vi "CRYGraph Wave Window.vi"() -> ()   [LabVIEW 2013]
uses:
  <vilib>/Utility/miscctls.llb/LVPoint32TypeDef.ctl
  Control/CRYFlag Cluster.ctl
  <vilib>/Utility/miscctls.llb/LVRowAndColumnTypeDef.ctl
  <vilib>/Utility/miscctls.llb/LVRectTypeDef.ctl
  CRYCurveLibrary/Global/CRYCurve Library Global.vi
  SubVI/CRYData View Global.vi
  SubVI/CRYMain Sub Window Global.vi
panel:
  out "LegendVScrollShow":bool=TRUE
  out "Legend Ref":refnum<vi>
  out "SelectedRow":i32[](array[numeric])
  in  "LoadFinish":bool
  in  "WhichKey":string
  out "KeyRepeatCount":i32
  in  "CursorMoveFinish":bool
  in  "ScaleFitY 2":bool
  in  "ScaleFitY":bool
  in  "ScaleFitX":bool
  in  "ToolbarUpdate":bool
  out "PropertyTab":string
  in  "OpenProperty":bool
  in  "PaletteShow":bool
  in  "FitPanes":bool
  out "PreviewScaleMax":dbl
  out "PreviewScaleMin":dbl
  out "PreviewCoords":T1
  in  "ScaleRange":bool
  out "Repaint Watermark":i32
  out "Event Name":string
  out "ReportDrop":bool
  out "DirectionKey":bool
  out "PreviewGraph Ref":refnum<vi>
  out "Graph Ref":refnum<vi>
  in  "AxisChange":bool
  in  "RemoveSome":bool
  out "ChildIntensityVI Ref":refnum<vi>
  in  "IntensityShow":bool
  out "ScaleMin":dbl
  out "ScaleMax":dbl
  out "ScrollTick Ref":refnum<vi>
  out "Scrollbar Ref":refnum<vi>
  in  "PreviewShow":bool
  in  "RemoveAll":bool
  in  "CursorColor":bool
  out "NewCursIdx":u32
  out "Test":string
  in  "OldCursIdx":u32
  out "Queue Name":string
  in  "StateOut":bool
  in  "Cursor Waves":string[](array[string])
  out "Cursor Coords":T1
  in  "CursorPlot":bool
  out "Cursor Ref":refnum<vi>
  in  "CursorShow":bool
  out "WaveGraph":cluster{"xo":dbl, "dx":dbl, dbl[]}[](graph)
  out "Title Name":string
  out "OldRow":i32
  out "TotalPlot":u32
  out "Graph Number":i32
  in  "stop":bool
  out "PreviewGraph":cluster{"xo":dbl, "dx":dbl, dbl[]}[](graph)
  in  "CursorEnabled":bool
  in  "Scrollbar":dbl(c297)
  in  "ScrollTick":dbl(slide) scale=0.0..1.0 scale format="%-#3.2p"
  in  "Cursor":string[][](table)
  in  "LegendShow":bool
  in  "ColorBox":u32(colorbox)
  in  "Legend":i32[](listbox)
  in  "GraphType":string
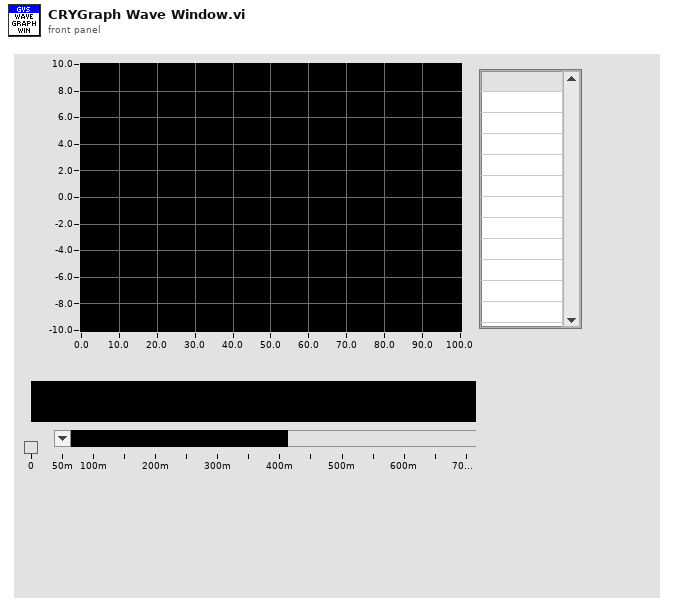
[diagram p1: front panel]
types:
  T1 = typedef "LVPoint32TypeDef.ctl" = cluster{"Horizontal":i32, "Vertical":i32}
  T2 = typedef "CRYFlag Cluster.ctl" = cluster{"LegendShow":bool, "CellClick":bool, "Total Number":bool, "ScaleFitX":bool, "ScaleFitY":bool, "MapModeX":u8, "MapModeY":u8, "CursorShow":bool, "MagnitudeShow":bool, "PreviewShow":bool, "CursorEnabled":bool, "IntensityShow":bool, "PaletteShow":bool, "PhaseShow":bool, "XYShow":bool, "FrequencyShow":bool, "LegendVScrollShow":bool, "FrequencyVScrollShow":bool}
  T3 = typedef "CRYGraph Event.ctl" = cluster{"EvenName":string, "TitleName":string, "GraphName":string, "GraphType":string, "Data":variant, "Queue Name":string, "DataView Number":i32}
  T4 = enum16{"No Scaling", "Scale All Objects", "Scale Single Object"}
  T5 = typedef "LVRowAndColumnTypeDef.ctl" = cluster{"Row":i32, "Column":i32}
  T6 = typedef "LVRectTypeDef.ctl" = cluster{"Left":i16, "Top":i16, "Right":i16, "Bottom":i16}
  T7 = typedef "LVBoundsTypeDef.ctl" = cluster{"Width":u32, "Height":u32}
  T8 = typedef "LVPositionTypeDef.ctl" = cluster{"Left":i32, "Top":i32}
  T9 = typedef "CRYWaveform Cluster.ctl" = cluster{"Waveform":cluster{"X0":dbl, "dX":dbl, "Y":sgl[]}, "X data":u16, "Y data":u16, "Y axis":u16, "X unit":string, "Y unit":string, "Y dB ref":dbl, "display Y":bool, "display X":bool, "Overload?":bool, "Test Info":string, "Step No.":i32, "Name":string, "protected":bool, "Sqc history":string[], "Signal Channel ID":i32, "Plot Settings":cluster{"Color":u32, "Interpolation":u8, "Point Style":u8, "Line Style":u8, "Point Color":u32, "Line Width":u8, "Bar Plot Style":u8, "Fill To":i16}, "AutoProtect":bool}
  T10 = typedef "LVRangeTypeDef.ctl" = cluster{"Minimum":dbl, "Maximum":dbl, "Increment":dbl, "Minor Increment":dbl, "Start":dbl}
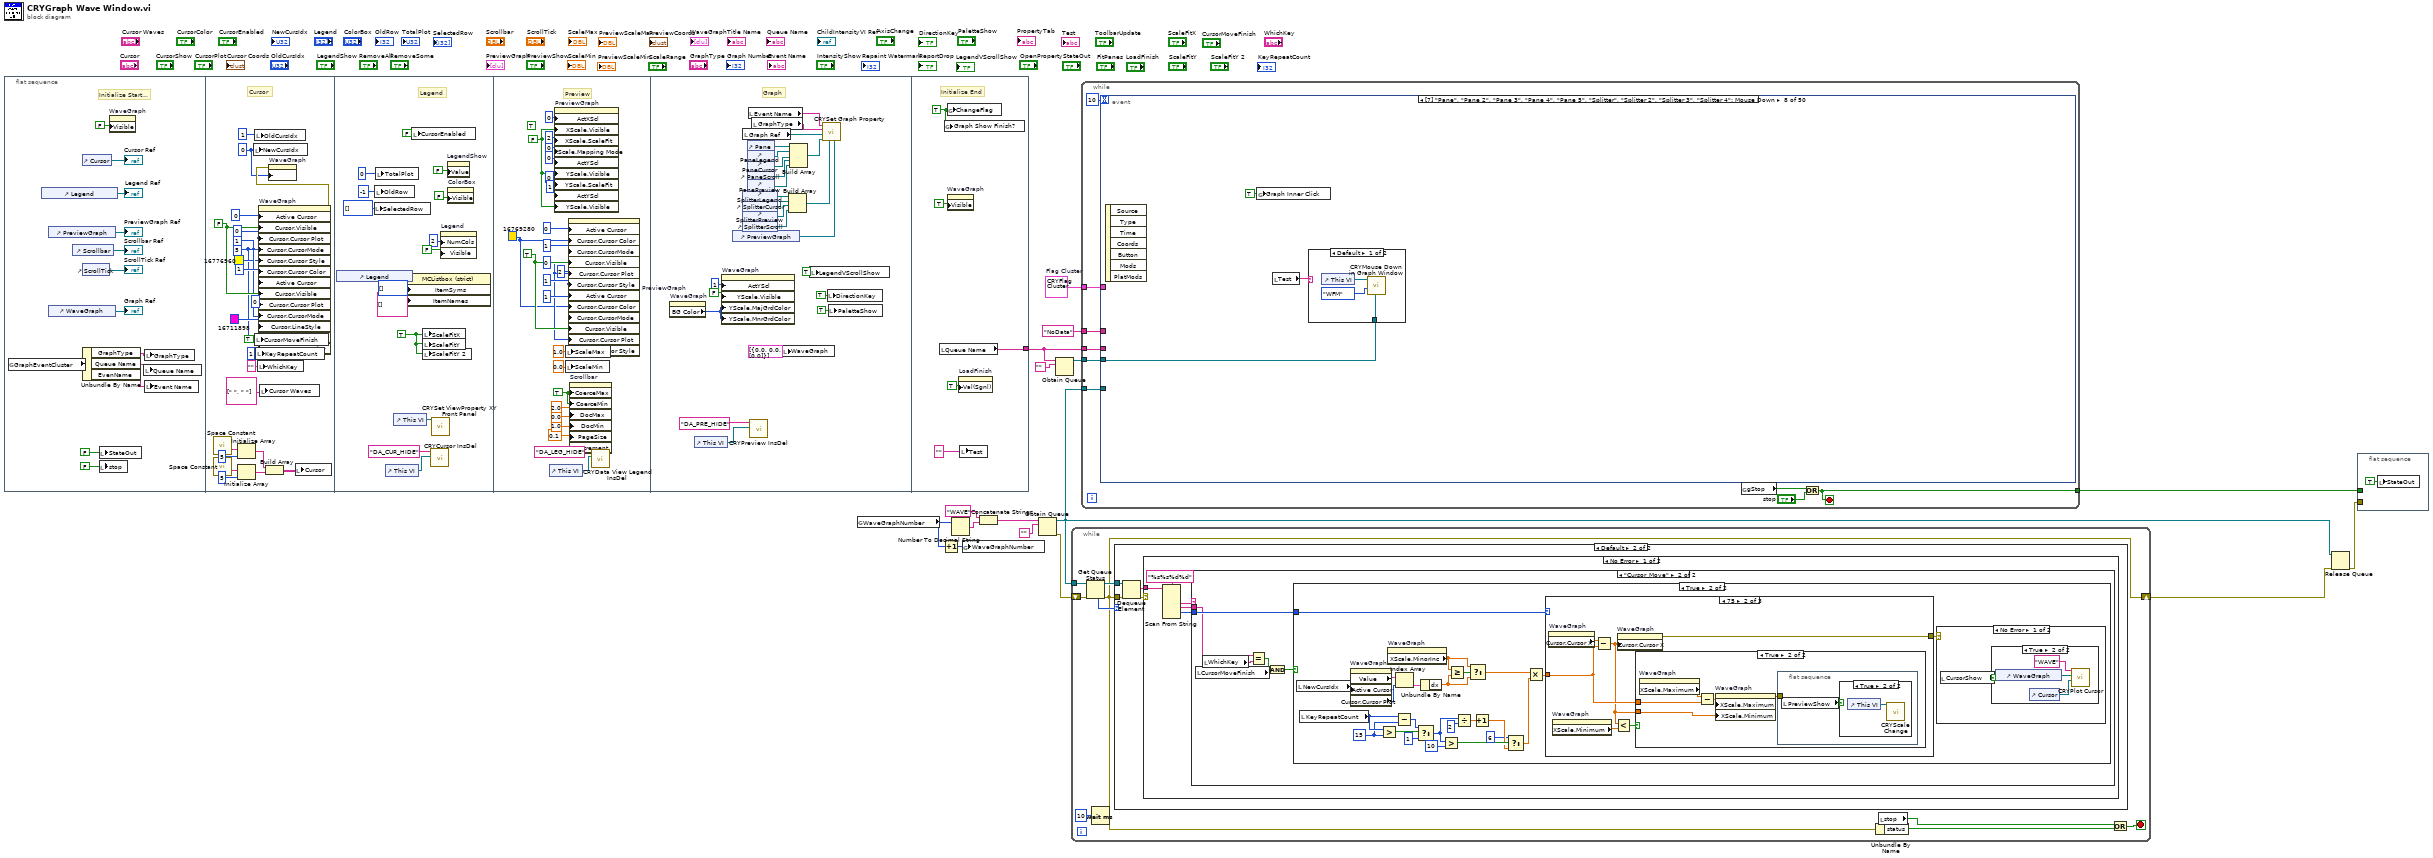
[diagram p0: block diagram]
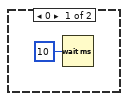
[diagram p2: hidden frame]
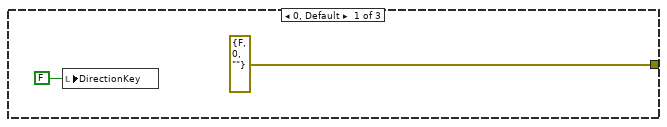
[diagram p7: hidden frame]
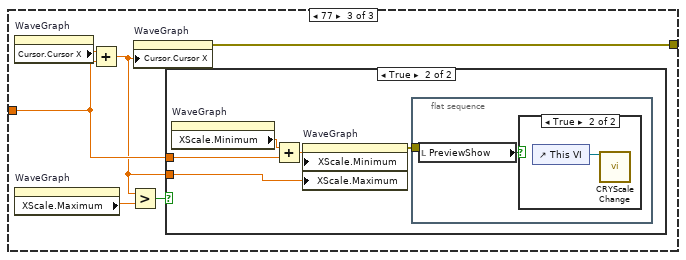
[diagram p10: hidden frame]
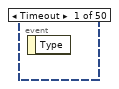
[diagram p14: hidden frame]
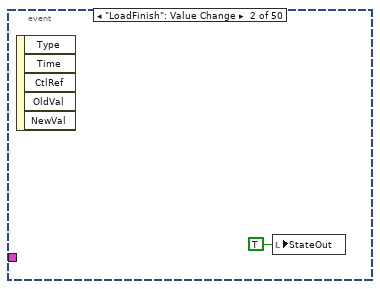
[diagram p15: hidden frame]
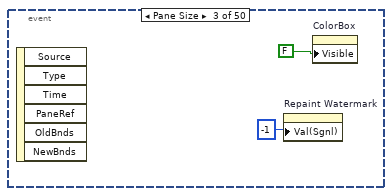
[diagram p16: hidden frame]
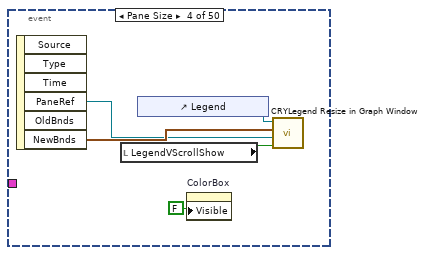
[diagram p17: hidden frame]
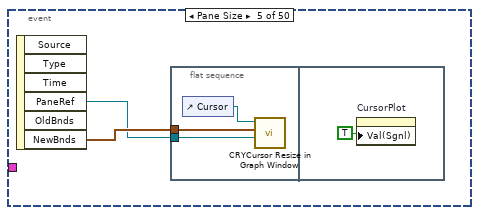
[diagram p18: hidden frame]
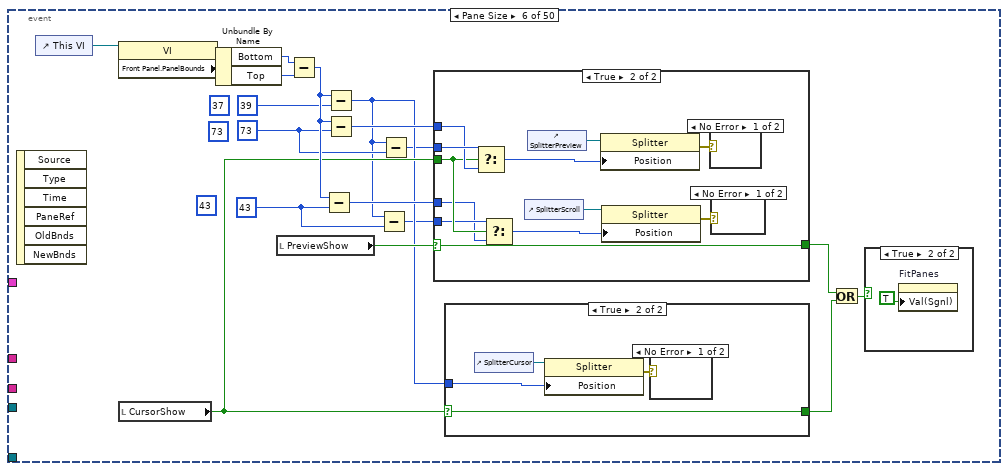
[diagram p19: hidden frame]
diagram:
  w14 = T2 {"LegendShow"=FALSE, "CellClick"=FALSE, "Total Number"=FALSE, "ScaleFitX"=FALSE, "ScaleFitY"=FALSE, "MapModeX"=0, "MapModeY"=0, "CursorShow"=FALSE, "MagnitudeShow"=FALSE, "PreviewShow"=FALSE, "CursorEnabled"=FALSE, "IntensityShow"=FALSE, "PaletteShow"=FALSE, "PhaseShow"=FALSE, "XYShow"=FALSE, "FrequencyShow"=FALSE, "LegendVScrollShow"=FALSE, "FrequencyVScrollShow"=FALSE}  # Flag Cluster
  n1 = flat-sequence {
    tunnel: [w118] -> w6
    frame #0 {
      # "Initialize Start..."
      n2 = global read "CRYData View Global.vi" "GraphEventCluster"() -> (w21:T3)
      n3 = control-ref of="Legend"() -> (→"Legend Ref":refnum<vi>)
      n4 = control-ref of="PreviewGraph"() -> (→"PreviewGraph Ref":refnum<vi>)
      n5 = control-ref of="WaveGraph"() -> (→"Graph Ref":refnum<vi>)
      n6 = control-ref of="Scrollbar"() -> (→"Scrollbar Ref":refnum<vi>)
      n7 = control-ref of="Cursor"() -> (→"Cursor Ref":refnum<vi>)
      n8 = control-ref of="ScrollTick"() -> (→"ScrollTick Ref":refnum<vi>)
      n9 = Unbundle By Name(w21) -> ("GraphType"=w19:string, "Queue Name"=w20:string, "EvenName"=w18:string)
      n10 = local write "StateOut"(FALSE ("StateOut")) -> ()
      n11 = local write "stop"(FALSE ("stop")) -> ()
      n12 = property on="WaveGraph" class="WFGraph (strict)"("Visible"=FALSE) -> ()  [unwired: 2 in, 2 out]
      n13 = local write "Queue Name"(w20) -> ()
      n14 = local write "GraphType"(w19) -> ()
      n15 = local write "Event Name"(w18) -> ()
    }
    frame #1 {
      w37 = u32 0 ("Active Cursor")
      w30 = u8 5 ("Cursor.Cursor Style")
      w39 = u32 1 ("Cursor.Cursor Mode")
      w40 = 0 ("Cursor.Cursor Plot")
      w41 = FALSE ("Cursor.Visible")
      # "Cursor"
      n16 = call <vilib>:"Space Constant.vi"() -> ("String"=w45:string)
      n17 = call <vilib>:"Space Constant.vi"() -> ("String"=w50:string)
      n18 = Initialize Array(w45, 5 ("dimension size")) -> (w47:string[])
      n19 = Initialize Array(w50, 5 ("dimension size")) -> (w51:string[])
      n20 = local write "NewCursIdx"(w37) -> ()
      n21 = local write "OldCursIdx"(u32 1 ("OldCursIdx")) -> ()
      n22 = local write "CursorMoveFinish"(TRUE ("CursorMove")) -> ()
      n23 = local write "KeyRepeatCount"(1 ("KeyRepeatCount")) -> ()
      n24 = local write "WhichKey"("" ("WhichKey")) -> ()
      n25 = property on="WaveGraph" class="WFGraph (strict)"("Active Cursor"=u32 0, "Cursor.Visible"=w41, "Cursor.Cursor Plot"=w40, "Cursor.CursorMode"=w39, "Cursor.Cursor Style"=w30, "Cursor.Cursor Color"=u32 16776960, "Active Cursor"=u32 1, "Cursor.Visible"=w41, "Cursor.Cursor Plot"=w40, "Cursor.CursorMode"=w39, "Cursor.LineStyle"=u8 0 ("Cursor.Line Style"), "Cursor.Cursor Style"=w30, "Cursor.Cursor Color"=u32 16711898) -> (error out=w38:errorcluster)  [unwired: 2 in, 1 out]
      n26 = local write "Cursor Waves"(string[] [" ", " "] ("Cursor Waves")) -> ()
      n27 = Build Array(w47, w51) -> (w48:string[][])
      n28 = property on="WaveGraph" class="WFGraph (strict)"(error in=w38, "Active Cursor"=w37) -> ()  [unwired: 1 in, 2 out]
      n29 = local write "Cursor"(w48) -> ()
    }
    frame #2 {
      w54 = TRUE ("ScaleFitX")
      # "Legend"
      n30 = control-ref of="Legend"() -> (w67:refnum<vi>)
      n31 = local write "SelectedRow"(i32[] [] ("SelectedRow")) -> ()
      n32 = local write "OldRow"(-1 ("OldRow 2")) -> ()
      n33 = local write "TotalPlot"(u32 0 ("TotalPlot")) -> ()
      n34 = control-ref of="This VI"() -> (w57:refnum<vi>)
      n35 = control-ref of="This VI"() -> (w55:refnum<vi>)
      n36 = property on="Property Node" class="MCListbox (strict)"(reference=w67, "ItemSyms"=i32[] [] ("Item Symbols"), "ItemNames"=string[][] [] ("Item Names")) -> ()  [unwired: 1 in, 2 out]
      n37 = local write "CursorEnabled"(FALSE ("CursorEnabled")) -> ()
      n38 = local write "ScaleFitX"(w54) -> ()
      n39 = local write "ScaleFitY"(w54) -> ()
      n40 = local write "ScaleFitY 2"(w54) -> ()
      n41 = call "CRYCursor InsDel.vi"("Graph VI Ref"=w57, "sAction"="DA_CUR_HIDE" ("Action Type")) -> ()  [unwired: 10 in]
      n42 = call "CRYSet ViewProperty XY  Front Panel.vi"("Vi Ref"=w55) -> ()  [unwired: 11 in]
      n43 = property on="Legend" class="MCListbox (strict)"("NumCols"=u32 2 ("Number of Columns"), "Visible"=FALSE) -> ()  [unwired: 2 in, 2 out]
      n44 = property on="LegendShow" class="Bool (strict)"("Value"=FALSE ("Visible")) -> ()  [unwired: 2 in, 2 out]
      n45 = property on="ColorBox" class="ColBox"("Visible"=FALSE) -> ()  [unwired: 2 in, 2 out]
    }
    frame #3 {
      w68 = u8 2 ("Cursor.Cursor Style")
      w71 = 0 ("Cursor.Cursor Plot")
      (unwired) TRUE ("X Scale.Visible")
      w69 = u32 16769280
      w79 = TRUE ("Cursor.Visible")
      w70 = FALSE ("X Scale.Visible")
      w91 = TRUE ("Coerce Maximum Value")
      # "Preview"
      n46 = control-ref of="This VI"() -> (w77:refnum<vi>)
      n47 = property on="PreviewGraph" class="WFGraph (strict)"("ActXScl"=0 ("Active X Scale"), "XScale.Visible"=w70, "XScale.ScaleFit"=u8 2 ("X Scale.Scale Fit"), "XScale.Mapping Mode"=u8 0 ("X Scale.Mapping Mode"), "ActYScl"=0 ("Active Y Scale"), "YScale.Visible"=w70, "YScale.ScaleFit"=u8 0 ("Y Scale.Scale Fit"), "ActYScl"=1 ("Active Y Scale"), "YScale.Visible"=w70) -> ()  [unwired: 2 in, 2 out]
      n48 = local write "ScaleMax"(1.0 ("ScaleMax")) -> ()
      n49 = local write "ScaleMin"(0.0 ("ScaleMin")) -> ()
      n50 = property on="PreviewGraph" class="WFGraph (strict)"("Active Cursor"=u32 0, "Cursor.Cursor Color"=w69, "Cursor.CursorMode"=u32 1 ("Cursor.Cursor Mode"), "Cursor.Visible"=w79, "Cursor.Cursor Plot"=w71, "Cursor.Cursor Style"=w68, "Active Cursor"=u32 1, "Cursor.Cursor Color"=w69, "Cursor.CursorMode"=u32 1 ("Cursor.Cursor Mode"), "Cursor.Visible"=w79, "Cursor.Cursor Plot"=w71, "Cursor.Cursor Style"=w68) -> ()  [unwired: 2 in, 2 out]
      n51 = property on="Scrollbar" class="Scroll (strict)"("CoerceMax"=w91, "CoerceMin"=w91, "DocMax"=2.0 ("Doc Max"), "DocMin"=0.0 ("Doc Min"), "PageSize"=1.0 ("Page Size"), "Increment"=0.1) -> ()  [unwired: 2 in, 2 out]
      n52 = call "CRYData View Legend InsDel.vi"("Graph VI Ref"=w77, "sAction"="DA_LEG_HIDE" ("Action Type")) -> ()  [unwired: 2 in, 8 out]
    }
    frame #4 {
      # "Graph"
      n53 = property on="WaveGraph" class="WFGraph (strict)"() -> ("BG Color"=w113:u32)  [unwired: 2 in, 2 out]
      n54 = control-ref of="This VI"() -> (w111:refnum<vi>)
      n55 = property on="WaveGraph" class="WFGraph (strict)"("ActYScl"=1 ("Active Y Scale"), "YScale.Visible"=FALSE ("Y Scale.Visible"), "YScale.MajGrdColor"=w113, "YScale.MnrGrdColor"=w113) -> ()  [unwired: 2 in, 2 out]
      n56 = control-ref of="PreviewGraph"() -> (w93:refnum<vi>)
      n57 = local read "Graph Ref"() -> (w108:refnum<vi>)
      n58 = control-ref of="SplitterLegend"() -> (w107:refnum<vi>)
      n59 = control-ref of="SplitterCursor"() -> (w106:refnum<vi>)
      n60 = control-ref of="SplitterPreview"() -> (w105:refnum<vi>)
      n61 = control-ref of="SplitterScroll"() -> (w104:refnum<vi>)
      n62 = control-ref of="Pane"() -> (w103:refnum<vi>)
      n63 = control-ref of="PaneLegend"() -> (w99:refnum<vi>)
      n64 = control-ref of="PaneCursor"() -> (w102:refnum<vi>)
      n65 = control-ref of="PaneScroll"() -> (w101:refnum<vi>)
      n66 = control-ref of="PanePreview"() -> (w100:refnum<vi>)
      n67 = local read "Event Name"() -> (w95:string)
      n68 = call "CRYPreview InsDel.vi"("Graph VI Ref"=w111, "sAction"="DA_PRE_HIDE" ("Action Type")) -> ()  [unwired: 10 in]
      n69 = local read "GraphType"() -> (w96:string)
      n70 = local write "WaveGraph"(cluster{"xo":dbl, "dx":dbl, dbl[]}[] [{"xo"=0.0, "dx"=0.0, [0.0]}] ("appended array")) -> ()
      n71 = Build Array(w107, w106, w105, w104) -> (w97:refnum<vi>[])
      n72 = Build Array(w103, w99, w102, w101, w100) -> (w98:refnum<vi>[])
      n73 = local write "LegendVScrollShow"(TRUE ("LegendVScrollShow")) -> ()
      n74 = call "CRYSet Graph Property.vi"("PreviewGraph Ref"=w93, "Splitters"=w97, "Panes"=w98, "Graph Ref"=w108, "Graph Type"=w96, "Event Name"=w95) -> ()  [unwired: 6 in]
      n75 = local write "DirectionKey"(TRUE ("ScanCode")) -> ()
      n76 = local write "PaletteShow"(TRUE ("PaletteShow")) -> ()
    }
    frame #5 {
      w120 = TRUE ("ChangeFlag")
      # "Initialize End"
      n77 = local read "Queue Name"() -> (w118:string)
      n78 = global write "CRYData View Global.vi" "Graph Show Finish?"(w120) -> ()
      n79 = global write "CRYData View Global.vi" "ChangeFlag"(w120) -> ()
      n80 = property on="WaveGraph" class="WFGraph (strict)"("Visible"=TRUE) -> ()  [unwired: 2 in, 2 out]
      n81 = property on="LoadFinish" class="Bool (strict)"("Val(Sgnl)"=TRUE ("Value (Signaling)")) -> ()  [unwired: 2 in, 2 out]
      n82 = local write "Test"("" ("Test")) -> ()
    }
  }
  n83 = global read "CRYCurve Library Global.vi" "WaveGraphNumber"() -> (w2:u32)
  n84 = Increment(x=w2) -> (x+1=w1:u32)
  n85 = Number To Decimal String(number=w2) -> (decimal integer string=w3:string)  [unwired: 1 in]
  n86 = global write "CRYCurve Library Global.vi" "WaveGraphNumber"(w1) -> ()
  n87 = Concatenate Strings("WAVE" ("YAxisTitle"), w3) -> (w5:string)
  n88 = Obtain Queue(name (unnamed)=w5, element data type="" ("Action Type")) -> (queue out=w7:refnum<queue>, error out=w11:errorcluster)  [unwired: 3 in, 1 out]
  n89 = Obtain Queue(name (unnamed)=w6, element data type="") -> (queue out=w16:refnum<queue>)  [unwired: 3 in, 2 out]
  n90 = while {
    tunnel: w7 -> [w127]
    shift-right: [w122] -> w10
    shift-left: w11 -> [w125]
    stop <- w128 stop-if-true
    n91 = Get Queue Status(queue=w127, error in (no error)=w125) -> (queue out=w126:refnum<queue>, error out=w122:errorcluster, # elements in queue=w123:i32)  [unwired: 6 out]
    n92 = Wait (ms)(milliseconds to wait=u32 10) -> ()  [unwired: 1 out]
    n93 = case shown="Default" w123 {
      tunnel: w126 -> [_ w134]
      tunnel: w122 -> [_ w133]
      frame 0 {
        n94 = Wait (ms)(milliseconds to wait=u32 10) -> ()  [unwired: 1 out]
      }
      frame Default {
        n95 = Dequeue Element(queue=w134, error in (no error)=w133) -> (element=w131:string, error out=w132:errorcluster)  [unwired: 3 out]
        n96 = case shown="No Error" w132 {
          tunnel: w131 -> [w138 _]
          frame No Error {
            n97 = Scan From String(format string="%s%s%d%d", input string=w138) -> (output 1=w136:string, output 2=w135:string, output 3=w137:i32)  [unwired: 2 in, 8 out]
            n98 = case shown="\"Cursor_Move\"" w136 {
              tunnel: w137 -> [_ w145]
              tunnel: w135 -> [_ w143]
              frame Default {
              }
              frame "Cursor_Move" {
                n99 = local read "CursorMoveFinish"() -> (w141:bool)
                n100 = local read "WhichKey"() -> (w144:string)
                n101 = Equal?(x=w143, y=w144) -> (x = y?=w142:bool)
                n102 = And(x=w142, y=w141) -> (x .and. y?=w140:bool)
                n103 = case shown="True" w140 {
                  tunnel: w145 -> [_ w161]
                  frame False {
                  }
                  frame True {
                    w154 = 15 ("y")
                    n104 = local read "NewCursIdx"() -> (w163:u32)
                    n105 = local read "KeyRepeatCount"() -> (w155:i32)
                    n106 = property on="WaveGraph" class="WFGraph (strict)"("Active Cursor"=w163) -> ("Value"=w162:cluster{"xo":dbl, "dx":dbl, dbl[]}[], "Cursor.Cursor Plot"=w164:i32)  [unwired: 2 in, 2 out]
                    n107 = Greater?(x=w155, y=w154) -> (0:w160:bool)
                    n108 = property on="WaveGraph" class="WFGraph (strict)"() -> ("XScale.MinorInc"=w166:dbl)  [unwired: 2 in, 2 out]
                    n109 = Index Array(array=w162, index=w164) -> (element=w168:cluster{"xo":dbl, "dx":dbl, dbl[]})
                    n110 = Subtract(x=w155, y=w154) -> (x-y=w156:i32)
                    n111 = Select(t=w156, s=w160, f=1) -> (s? t:f=w149:i32)
                    n112 = Unbundle By Name(w168) -> ("dx"=w169:dbl)
                    n113 = Greater?(x=w149, y=10) -> (0:w153:bool)
                    n114 = Greater Or Equal?(x=w166, y=w169) -> (x >= y?=w165:bool)
                    n115 = Divide(x=w149, y=2 ("x")) -> (x/y=w150:dbl)
                    n116 = Select(t=w166, s=w165, f=w169) -> (s? t:f=w159:dbl)
                    n117 = Increment(x=w150) -> (x+1=w147:dbl)
                    n118 = Select(t=6 ("x"), s=w153, f=w147) -> (s? t:f=w151:dbl)
                    n119 = Multiply(x=w159, y=w151) -> (x*y=w158:dbl)
                    n120 = case shown="75" w161 {
                      tunnel: w158 -> [_ w177 w190]
                      tunnel: [errorcluster {"status"=FALSE, "code"=0, "source"=""} ("error out") w181 w194] -> w167
                      frame 0, Default {
                        n121 = local write "DirectionKey"(FALSE ("ScanCode")) -> ()
                      }
                      frame 75 {
                        n122 = property on="WaveGraph" class="WFGraph (strict)"() -> ("Cursor.Cursor X"=w180:dbl)  [unwired: 2 in, 2 out]
                        n123 = property on="WaveGraph" class="WFGraph (strict)"() -> ("XScale.Minimum"=w179:dbl)  [unwired: 2 in, 2 out]
                        n124 = Subtract(x=w180, y=w177) -> (x-y=w176:dbl)
                        n125 = Less?(x=w176, y=w179) -> (x < y?=w178:bool)
                        n126 = property on="WaveGraph" class="WFGraph (strict)"("Cursor.Cursor X"=w176) -> (error out=w181:errorcluster)  [unwired: 2 in, 1 out]
                        n127 = case shown="True" w178 {
                          tunnel: w176 -> [_ w186]
                          tunnel: w177 -> [_ w183]
                          frame False {
                          }
                          frame True {
                            n128 = property on="WaveGraph" class="WFGraph (strict)"() -> ("XScale.Maximum"=w184:dbl)  [unwired: 2 in, 2 out]
                            n129 = Subtract(x=w184, y=w183) -> (x-y=w185:dbl)
                            n130 = property on="WaveGraph" class="WFGraph (strict)"("XScale.Maximum"=w185, "XScale.Minimum"=w186) -> (error out=w182:errorcluster)  [unwired: 2 in, 1 out]
                            n131 = flat-sequence {
                              tunnel: w182 -> [_]
                              frame #0 {
                                n132 = local read "PreviewShow"() -> (w187:bool)
                                n133 = case shown="True" w187 {
                                frame False {
                                }
                                frame True {
                                n134 = control-ref of="This VI"() -> (w188:refnum<vi>)
                                n135 = call "CRYScale Change.vi"("Graph VI Ref"=w188) -> ()  [unwired: 11 in]
                                }
                                }
                              }
                            }
                          }
                        }
                      }
                      frame 77 {
                        n136 = property on="WaveGraph" class="WFGraph (strict)"() -> ("Cursor.Cursor X"=w193:dbl)  [unwired: 2 in, 2 out]
                        n137 = property on="WaveGraph" class="WFGraph (strict)"() -> ("XScale.Maximum"=w192:dbl)  [unwired: 2 in, 2 out]
                        n138 = Add(x=w193, y=w190) -> (x+y=w189:dbl)
                        n139 = Greater?(x=w189, y=w192) -> (0:w191:bool)
                        n140 = property on="WaveGraph" class="WFGraph (strict)"("Cursor.Cursor X"=w189) -> (error out=w194:errorcluster)  [unwired: 2 in, 1 out]
                        n141 = case shown="True" w191 {
                          tunnel: w189 -> [_ w199]
                          tunnel: w190 -> [_ w197]
                          frame False {
                          }
                          frame True {
                            n142 = property on="WaveGraph" class="WFGraph (strict)"() -> ("XScale.Minimum"=w196:dbl)  [unwired: 2 in, 2 out]
                            n143 = Add(x=w196, y=w197) -> (x+y=w198:dbl)
                            n144 = property on="WaveGraph" class="WFGraph (strict)"("XScale.Minimum"=w198, "XScale.Maximum"=w199) -> (error out=w195:errorcluster)  [unwired: 2 in, 1 out]
                            n145 = flat-sequence {
                              tunnel: w195 -> [_]
                              frame #0 {
                                n146 = local read "PreviewShow"() -> (w200:bool)
                                n147 = case shown="True" w200 {
                                frame False {
                                }
                                frame True {
                                n148 = control-ref of="This VI"() -> (w201:refnum<vi>)
                                n149 = call "CRYScale Change.vi"("Graph VI Ref"=w201) -> ()  [unwired: 11 in]
                                }
                                }
                              }
                            }
                          }
                        }
                      }
                    }
                    n150 = case shown="No Error" w167 {
                      frame No Error {
                        n151 = local read "CursorShow"() -> (w170:bool)
                        n152 = case shown="True" w170 {
                          frame False {
                          }
                          frame True {
                            n153 = control-ref of="WaveGraph"() -> (w173:refnum<vi>)
                            n154 = control-ref of="Cursor"() -> (w172:refnum<vi>)
                            n155 = call "CRYPlot Cursor.vi"("Cursor Ref"=w172, "Graph Ref"=w173, "Graph Type"="WAVE") -> ()  [unwired: 9 in]
                          }
                        }
                      }
                      frame Error {
                      }
                    }
                  }
                }
              }
            }
          }
          frame Error {
          }
        }
      }
    }
    n156 = Unbundle By Name(w122) -> ("status"=w129:bool)
    n157 = local read "stop"() -> (w121:bool)
    n158 = Or(x=w121, y=w129) -> (x .or. y?=w128:bool)
  }
  n159 = while {
    tunnel: w16 -> [w210]
    tunnel: w14 -> [w208]
    tunnel: "NoData" ("input 2") -> [w205]
    tunnel: w6 -> [w204]
    tunnel: [w203] -> w12
    tunnel: w7 -> [w202]
    stop <- w203 stop-if-true
    n160 = event shown="[7] \"Pane\", \"Pane 2\", \"Pane 3\", \"Pane 4\", \"Pane 5\", \"Splitter\", \"Splitter 2\", \"Splitter 3\", \"Splitter 4\": Mouse Down" {
      selector: _ -> [_ _ _ _ _ _ _ _ _ _ _ _ _ _ _ _ _ _ _ _ _ _ _ _ _ _ _ _ _ _ _ _ _ _ _ _ _ _ _ _ _ _ _ _ _ _ _ _ _ _]
      dyn-events: _ -> [_ _ _ _ _ _ _ _ _ _ _ _ _ _ _ _ _ _ _ _ _ _ _ _ _ _ _ _ _ _ _ _ _ _ _ _ _ _ _ _ _ _ _ _ _ _ _ _ _ _]
      timeout: 10 -> [_ _ _ _ _ _ _ _ _ _ _ _ _ _ _ _ _ _ _ _ _ _ _ _ _ _ _ _ _ _ _ _ _ _ _ _ _ _ _ _ _ _ _ _ _ _ _ _ _ _]
      tunnel: w210 -> [_ _ _ _ _ _ _ w280 _ w313 _ w468 _ w521 _ w572 _ _ _ _ _ _ _ _ _ _ _ _ _ _ w801 _ _ _ _ _ w992 _ _ w1005 _ _ _ _ _ _ _ _ _ _]
      tunnel: w208 -> [_ _ _ _ _ _ _ _ w297 _ w446 _ w506 _ w565 _ _ _ _ _ _ _ _ _ _ _ _ _ _ _ _ _ _ _ _ _ _ _ _ _ _ _ _ _ _ _ _ _ _ _]
      tunnel: w205 -> [_ _ _ _ _ _ _ _ _ w315 _ _ _ w520 _ _ _ _ _ _ _ _ _ _ _ _ _ _ _ _ _ _ _ _ _ _ _ _ _ _ _ _ _ _ _ _ _ _ _ _]
      tunnel: w204 -> [_ _ _ _ _ _ _ _ w290 w314 _ _ _ _ _ _ _ _ _ _ _ _ _ _ _ _ _ _ _ _ _ _ _ _ _ _ _ _ _ _ _ _ _ _ _ _ _ _ _ _]
      tunnel: w202 -> [_ _ _ _ _ _ _ _ _ _ _ _ _ _ _ _ _ w649 w668 w683 _ _ _ _ _ _ _ _ _ _ _ _ _ _ _ _ _ _ _ _ _ _ _ _ _ _ _ _ _ _]
      event Timeout {
        n161 = event-data() -> ()  [unwired: 2 out]
      }
      event "LoadFinish": Value Change {
        n162 = event-data() -> ()  [unwired: 6 out]
        n163 = local write "StateOut"(TRUE ("StateOut")) -> ()
      }
      event Pane Size {
        n164 = event-data() -> ()  [unwired: 7 out]
        n165 = property on="Repaint Watermark" class="DigNum (strict)"("Val(Sgnl)"=-1 ("y")) -> ()  [unwired: 2 in, 2 out]
        n166 = property on="ColorBox" class="ColBox"("Visible"=FALSE) -> ()  [unwired: 2 in, 2 out]
      }
      event Pane Size {
        n167 = event-data() -> ("PaneRef"=w216:refnum<vi>, "NewBnds"=w217:T6)  [unwired: 5 out]
        n168 = local read "LegendVScrollShow"() -> (w214:bool)
        n169 = control-ref of="Legend"() -> (w215:refnum<vi>)
        n170 = property on="ColorBox" class="ColBox"("Visible"=FALSE) -> ()  [unwired: 2 in, 2 out]
        n171 = call "CRYLegend Resize in Graph Window.vi"("VScrollShow"=w214, "Pane Ref"=w216, "input cluster"=w217, "Legend"=w215) -> ()  [unwired: 8 out]
      }
      event Pane Size {
        n172 = event-data() -> ("PaneRef"=w219:refnum<vi>, "NewBnds"=w220:T6)  [unwired: 5 out]
        n173 = flat-sequence {
          tunnel: w220 -> [w223]
          tunnel: w219 -> [w221]
          frame #0 {
            n174 = control-ref of="Cursor"() -> (w222:refnum<vi>)
            n175 = call "CRYCursor Resize in Graph Window.vi"("Pane Ref"=w221, "input cluster"=w223, "Graph Cursor Ref"=w222) -> ()  [unwired: 9 in]
          }
          frame #1 {
            n176 = property on="CursorPlot" class="Bool (strict)"("Val(Sgnl)"=TRUE ("Value (Signaling)")) -> ()  [unwired: 2 in, 2 out]
          }
        }
      }
      event Pane Size {
        (unwired) 43
        (unwired) 73
        (unwired) 37
        w227 = 43
        w229 = 73
        n177 = event-data() -> ()  [unwired: 7 out]
        n178 = control-ref of="This VI"() -> (w240:refnum<vi>)
        n179 = property class="VI"(reference=w240) -> ("Front Panel.PanelBounds"=w239:T6)  [unwired: 1 in, 2 out]
        n180 = local read "CursorShow"() -> (w230:bool)
        n181 = Unbundle By Name(w239) -> ("Bottom"=w242:i16, "Top"=w241:i16)
        n182 = local read "PreviewShow"() -> (w237:bool)
        n183 = Subtract(x=w242, y=w241) -> (x-y=w238:i16)
        n184 = Subtract(x=w238, y=w227) -> (x-y=w235:i32)
        n185 = Subtract(x=w238, y=39) -> (x-y=w228:i32)
        n186 = Subtract(x=w238, y=w229) -> (x-y=w236:i32)
        n187 = Subtract(x=w228, y=w227) -> (x-y=w225:i32)
        n188 = Subtract(x=w228, y=w229) -> (x-y=w226:i32)
        n189 = case shown="True" w237 {
          selector: w237 -> [w244 w252]
          tunnel: w236 -> [_ w250]
          tunnel: w235 -> [_ w246]
          tunnel: [w244 w252] -> w234
          tunnel: w230 -> [_ w248]
          tunnel: w226 -> [_ w251]
          tunnel: w225 -> [_ w247]
          frame False {
          }
          frame True {
            n190 = Select(t=w251, s=w248, f=w250) -> (s? t:f=w249:i32)
            n191 = Select(t=w247, s=w248, f=w246) -> (s? t:f=w245:i32)
            n192 = control-ref of="SplitterScroll"() -> (w255:refnum<vi>)
            n193 = control-ref of="SplitterPreview"() -> (w256:refnum<vi>)
            n194 = property class="Splitter"(reference=w256, "Position"=w249) -> (error out=w254:errorcluster)  [unwired: 1 in, 1 out]
            n195 = property class="Splitter"(reference=w255, "Position"=w245) -> (error out=w253:errorcluster)  [unwired: 1 in, 1 out]
            n196 = case shown="No Error" w254 {
              frame No Error {
              }
              frame Error {
              }
            }
            n197 = case shown="No Error" w253 {
              frame No Error {
              }
              frame Error {
              }
            }
          }
        }
        n198 = case shown="True" w230 {
          selector: w230 -> [w257 w258]
          tunnel: w228 -> [_ w260]
          tunnel: [w257 w258] -> w233
          frame False {
          }
          frame True {
            n199 = control-ref of="SplitterCursor"() -> (w261:refnum<vi>)
            n200 = property class="Splitter"(reference=w261, "Position"=w260) -> (error out=w259:errorcluster)  [unwired: 1 in, 1 out]
            n201 = case shown="No Error" w259 {
              frame No Error {
              }
              frame Error {
              }
            }
          }
        }
        n202 = Or(x=w234, y=w233) -> (x .or. y?=w232:bool)
        n203 = case shown="True" w232 {
          frame False {
          }
          frame True {
            n204 = property on="FitPanes" class="Bool (strict)"("Val(Sgnl)"=TRUE ("Value (Signaling)")) -> ()  [unwired: 2 in, 2 out]
          }
        }
      }
      event "FitPanes": Value Change {
        n205 = event-data() -> ()  [unwired: 7 out]
        n206 = local read "PreviewShow"() -> (w262:bool)
        n207 = local read "CursorShow"() -> (w263:bool)
        n208 = case shown="True" w262 {
          frame False {
          }
          frame True {
            n209 = control-ref of="PreviewGraph"() -> (w269:refnum<vi>)
            n210 = control-ref of="Scrollbar"() -> (w268:refnum<vi>)
            n211 = control-ref of="ScrollTick"() -> (w267:refnum<vi>)
            n212 = invoke class="WFGraph (strict)" method="FitControlToPane"(reference=w269) -> (error out=w266:errorcluster)  [unwired: 2 in, 2 out]
            n213 = invoke class="Scroll (strict)" method="FitControlToPane"(reference=w268) -> (error out=w265:errorcluster)  [unwired: 2 in, 2 out]
            n214 = invoke class="Slide (strict)" method="FitControlToPane"(reference=w267) -> (error out=w264:errorcluster)  [unwired: 2 in, 2 out]
            n215 = flat-sequence {
              tunnel: w265 -> [_]
              tunnel: w264 -> [_]
              frame #0 {
                n216 = control-ref of="PaneScroll"() -> (w273:refnum<vi>)
                n217 = invoke class="Pane" method="Set Scaling"(reference=w273, "ScalingMode"=T4."No Scaling" ("Scaling Mode")) -> ()  [unwired: 3 in, 5 out]
              }
            }
            n218 = control-ref of="PanePreview"() -> (w271:refnum<vi>)
            n219 = invoke class="Pane" method="Set Scaling"(reference=w271, error in=w266, "ScalingMode"=T4."No Scaling" ("Scaling Mode")) -> ()  [unwired: 2 in, 5 out]
          }
        }
        n220 = case shown="True" w263 {
          frame False {
          }
          frame True {
            n221 = control-ref of="Cursor"() -> (w277:refnum<vi>)
            n222 = invoke class="Tbl (strict)" method="FitControlToPane"(reference=w277) -> (error out=w275:errorcluster)  [unwired: 2 in, 2 out]
            n223 = control-ref of="PaneCursor"() -> (w276:refnum<vi>)
            n224 = invoke class="Pane" method="Set Scaling"(reference=w276, error in=w275, "ScalingMode"=T4."No Scaling" ("Scaling Mode")) -> ()  [unwired: 2 in, 5 out]
          }
        }
      }
      event Mouse Down {
        n225 = event-data() -> ()  [unwired: 8 out]
        n226 = global write "CRYCurve Library Global.vi" "Graph Inner Click"(TRUE ("Graph Inner Click")) -> ()
        n227 = local read "Test"() -> (w279:string)
        n228 = case shown="Default" w279 {
          tunnel: w280 -> [w283 _]
          frame Default {
            n229 = control-ref of="This VI"() -> (w281:refnum<vi>)
            n230 = call "CRYMouse Down in Graph Window.vi"("Queue"=w283, "Selected Type"=enum16{"Curves", "Values", "Results", "WFM"}."WFM" ("Type"), "pGraph VI In"=w281) -> ()  [unwired: 3 in, 6 out]
          }
          frame "Test" {
          }
        }
      }
      event Shortcut Menu Activation? {
        n231 = event-data() -> ("MenuRef"=w299:refnum<k9>)  [unwired: 7 out]
        n232 = property on="WaveGraph" class="WFGraph (strict)" props=["XScale", "ScaleFit", "YScale", "ScaleFit", "XScale", "Mapping Mode", "YScale", "Mapping Mode"]() -> ("XScale.Mapping Mode"=w295:u8, "YScale.Mapping Mode"=w294:u8)  [unwired: 2 in, 4 out]
        n233 = local read "CursorEnabled"() -> (w292:bool)
        n234 = local read "LegendShow"() -> (w298:bool)
        n235 = local read "PreviewShow"() -> (w291:bool)
        n236 = local read "PaletteShow"() -> (w286:bool)
        n237 = local read "CursorShow"() -> (w293:bool)
        n238 = local read "ScaleFitX"() -> (w285:bool)
        n239 = local read "ScaleFitY"() -> (w284:bool)
        n240 = Bundle By Name(cluster=w297, "LegendShow"=w298, "ScaleFitX"=w285, "ScaleFitY"=w284, "MapModeX"=w295, "MapModeY"=w294, "CursorShow"=w293, "PreviewShow"=w291, "CursorEnabled"=w292, "PaletteShow"=w286) -> (w296:T2)
        n241 = local read "Test"() -> (w287:string)
        n242 = case shown="Default" w287 {
          tunnel: w290 -> [_ w305]
          tunnel: ["" ("sData Out") w304] -> w289
          tunnel: [TRUE ("bResult Out") w303] -> w288
          frame "Test" {
          }
          frame Default {
            n243 = local read "Graph Number"() -> (w302:i32)
            n244 = call "CRYGraph View Socket Client.vi"("sOption"="MENUOPTION", "nData"=w302, "sData"=w305, "sAction"="GET_GRAPHDATA") -> ("bResult Out"=w303:bool, "sData Out"=w304:string)  [unwired: 4 in, 2 out]
          }
        }
        n245 = case shown="True" w288 {
          tunnel: w299 -> [_ w312]
          tunnel: w296 -> [_ w310]
          tunnel: w289 -> [_ w309]
          frame False {
          }
          frame True {
            n246 = control-ref of="This VI"() -> (w308:refnum<vi>)
            n247 = call "CRYGraph Window Menu.vi"("MenuOption"=w309, "pGraph VI"=w308, "Flag Cluster"=w310, "Type"="WAVE", "Runtime Menu Ref In"=w312) -> ()  [unwired: 7 out]
          }
        }
        n248 = event-data() -> ()  [unwired: 1 in, 2 out]
      }
      event Shortcut Menu Selection (User) {
        n249 = event-data() -> ("ItemTag"=w316:string)  [unwired: 1 out]
        n250 = case shown="\"DA_EXPORT_EXCEL\"" w316 {
          selector: w316 -> [w318 _ w406 _ w442 _]
          tunnel: w315 -> [_ _ w400 _ _ _]
          tunnel: w314 -> [_ _ _ w431 _ _]
          tunnel: w313 -> [_ _ w398 _ _ _]
          frame "DA_SCALE_X_A", "DA_SCALE_X_L", "DA_SCALE_Y_A", "DA_SCALE_Y_L" {
            n251 = case shown="\"DA_SCALE_X_A\", Default" w318 {
              selector: w318 -> [w322 w369 w373 w394]
              tunnel: [w322 w369 w373 w394] -> w317
              frame "DA_SCALE_X_A", Default {
                n252 = local read "ScaleFitX"() -> (w321:bool)
                n253 = Not(x=w321) -> (.not. x?=w320:bool)
                n254 = Select(t=u8 2, s=w320, f=u8 0) -> (s? t:f=w323:u8)
                n255 = local write "ScaleFitX"(w320) -> ()
                n256 = property on="WaveGraph" class="WFGraph (strict)"("XScale.ScaleFit"=w323) -> (error out=w324:errorcluster)  [unwired: 2 in, 1 out]
                n257 = case shown="2" w323 {
                  tunnel: w324 -> [_ _]
                  frame Default {
                  }
                  frame 2 {
                    n258 = property on="PreviewGraph" class="WFGraph (strict)"() -> ("XScale.Maximum"=w336:dbl, "XScale.Minimum"=w330:dbl)  [unwired: 2 in, 2 out]
                    n259 = property on="WaveGraph" class="WFGraph (strict)"() -> ("XScale.Maximum"=w355:dbl, "XScale.Minimum"=w356:dbl)  [unwired: 2 in, 2 out]
                    n260 = Greater?(x=w330, y=w356) -> (0:w357:bool)
                    n261 = Less?(x=w336, y=w355) -> (x < y?=w354:bool)
                    n262 = Subtract(x=w336, y=w330) -> (x-y=w335:dbl)
                    n263 = Select(t=w336, s=w354, f=w355) -> (s? t:f=w331:dbl)
                    n264 = Select(t=w330, s=w357, f=w356) -> (s? t:f=w332:dbl)
                    n265 = Subtract(x=w332, y=w330) -> (x-y=w329:dbl)
                    n266 = Subtract(x=w331, y=w330) -> (x-y=w328:dbl)
                    n267 = property on="PreviewGraph" class="WFGraph (strict)"("Active Cursor"=u32 0, "Cursor.Cursor X"=w332, "Active Cursor"=u32 1, "Cursor.Cursor X"=w331) -> (error out=w353:errorcluster)  [unwired: 2 in, 1 out]
                    n268 = Divide(x=w329, y=w335) -> (x/y=w333:dbl)
                    n269 = Divide(x=w328, y=w335) -> (x/y=w334:dbl)
                    n270 = property on="Scrollbar" class="Scroll (strict)"() -> ("DocMax"=w342:dbl, "PageSize"=w348:dbl)  [unwired: 2 in, 2 out]
                    n271 = Subtract(x=w333, y=w334) -> (x-y=w340:dbl)
                    n272 = flat-sequence {
                      tunnel: w353 -> [_]
                      frame #0 {
                        n273 = control-ref of="This VI"() -> (w359:refnum<vi>)
                        n274 = call "CRYPlot Wave Graph Preview.vi"("sOption"="Move", "Graph VI Ref"=w359) -> ()  [unwired: 10 in]
                      }
                    }
                    n275 = Divide(x=w348, y=w340) -> (x/y=w339:dbl)
                    n276 = local read "ScaleMax"() -> (w338:dbl)
                    n277 = local read "ScaleMin"() -> (w337:dbl)
                    n278 = Add(x=w342, y=w339) -> (x+y=w341:dbl)
                    n279 = property on="Scrollbar" class="Scroll (strict)"("DocMin"=w341) -> ("DocMax"=w350:dbl, "DocMin"=w349:dbl)  [unwired: 2 in, 2 out]
                    n280 = Subtract(x=w338, y=w337) -> (x-y=w327:dbl)
                    n281 = Subtract(x=w333, y=w337) -> (x-y=w343:dbl)
                    n282 = Subtract(x=w350, y=w349) -> (x-y=w344:dbl)
                    n283 = Multiply(x=w343, y=w344) -> (x*y=w345:dbl)
                    n284 = Divide(x=w345, y=w327) -> (x/y=w346:dbl)
                    n285 = Add(x=w346, y=w349) -> (x+y=w347:dbl)
                    n286 = property on="Scrollbar" class="Scroll (strict)"("Value"=w347) -> ()  [unwired: 2 in, 2 out]
                  }
                }
              }
              frame "DA_SCALE_Y_A" {
                n287 = local read "ScaleFitY 2"() -> (w361:bool)
                n288 = local read "ScaleFitY"() -> (w363:bool)
                n289 = Not(x=w363) -> (.not. x?=w362:bool)
                n290 = Not(x=w361) -> (.not. x?=w360:bool)
                n291 = Select(t=u8 2, s=w362, f=u8 0) -> (s? t:f=w370:u8)
                n292 = Select(t=u8 2, s=w360, f=u8 0) -> (s? t:f=w366:u8)
                n293 = property on="WaveGraph" class="WFGraph (strict)"("ActYScl"=0 ("Active Y Scale"), "YScale.ScaleFit"=w370) -> ()  [unwired: 2 in, 2 out]
                n294 = property on="WaveGraph" class="WFGraph (strict)"("ActYScl"=1 ("Active Y Scale"), "YScale.ScaleFit"=w366) -> ()  [unwired: 2 in, 2 out]
                n295 = local write "ScaleFitY"(w362) -> ()
                n296 = local write "ScaleFitY 2"(w360) -> ()
              }
              frame "DA_SCALE_X_L" {
                n297 = property on="WaveGraph" class="WFGraph (strict)"() -> ("XScale.Mapping Mode"=w374:u8)  [unwired: 2 in, 2 out]
                n298 = Equal?(x=w374, y=u8 0) -> (x = y?=w379:bool)
                n299 = Select(t=u8 1, s=w379, f=u8 0) -> (s? t:f=w375:u8)
                n300 = property on="WaveGraph" class="WFGraph (strict)"("XScale.Mapping Mode"=w375) -> ()  [unwired: 2 in, 2 out]
              }
              frame "DA_SCALE_Y_L" {
                n301 = property on="WaveGraph" class="WFGraph (strict)"("ActYScl"=0 ("Active Y Scale")) -> ("YScale.Mapping Mode"=w383:u8)  [unwired: 2 in, 2 out]
                n302 = property on="WaveGraph" class="WFGraph (strict)"("ActYScl"=1 ("Active Y Scale")) -> ("YScale.Mapping Mode"=w390:u8)  [unwired: 2 in, 2 out]
                n303 = Equal To 0?(x=w383) -> (x = 0?=w386:bool)
                n304 = Equal To 0?(x=w390) -> (x = 0?=w387:bool)
                n305 = Select(t=u8 1, s=w386, f=u8 0) -> (s? t:f=w382:u8)
                n306 = Select(t=u8 1, s=w387, f=u8 0) -> (s? t:f=w391:u8)
                n307 = property on="WaveGraph" class="WFGraph (strict)"("ActYScl"=0 ("Active Y Scale"), "YScale.Mapping Mode"=w382) -> ()  [unwired: 2 in, 2 out]
                n308 = property on="WaveGraph" class="WFGraph (strict)"("ActYScl"=1 ("Active Y Scale"), "YScale.Mapping Mode"=w391) -> ()  [unwired: 2 in, 2 out]
              }
            }
            n309 = case shown="\"DA_SCALE_X_A\", \"DA_SCALE_Y_A\"" w317 {
              frame "False", Default {
              }
              frame "DA_SCALE_X_A", "DA_SCALE_Y_A" {
                n310 = property on="ToolbarUpdate" class="Bool (strict)"("Val(Sgnl)"=TRUE ("Value (Signaling)")) -> ()  [unwired: 2 in, 2 out]
              }
            }
          }
          frame "DA_EXPORT_EXCEL" {
            w396 = enum16{"Curves", "Values", "Results", "WFM"}."WFM" ("Type")
            n311 = control-ref of="Legend"() -> (w395:refnum<vi>)
            n312 = call "CRYGet Graph Data in Graph.vi"("Legend Refnum"=w395, "Type In"=w396) -> ("Rows"=w397:i32[])  [unwired: 2 in, 7 out]
            n313 = call "CRYExport to Excel.vi"("Rows"=w397, "Type"=w396) -> ()  [unwired: 2 in, 8 out]
          }
          frame Default {
            n314 = Search/Split String(string=w406, search string/char (-)="#") -> (substring before match=w401:string, match + rest of string=w404:string)  [unwired: 2 out]
            n315 = call "CRYPreUpdate Sequence.vi"("EventName"="CurLibUpdate") -> ()  [unwired: 15 in]
            n316 = Decimal String To Number(string=w404, offset=1) -> (number=w402:i32)  [unwired: 2 out]
            n317 = case shown="0, Default" w402 {
              selector: w402 -> [_ w419]
              tunnel: w401 -> [w408 w421]
              tunnel: w400 -> [_ _]
              tunnel: w398 -> [w413 w417]
              frame 0, Default {
                n318 = Equal?(x="DA_EXPORT_DOCUMENT" ("y"), y=w408) -> (x = y?=w410:bool)
                n319 = Select(t="ADD_DOC", s=w410, f=w408) -> (s? t:f=w409:string)
                n320 = local read "Graph Number"() -> (w414:i32)
                n321 = local read "GraphType"() -> (w407:string)
                n322 = Format Into String(w409, w407, w414, 0 ("input 3")) -> (resulting string=w415:string)  [unwired: 3 in, 1 out]
                n323 = Enqueue Element(queue=w413, element=w415) -> ()  [unwired: 1 in, 4 out]
              }
              frame 1..10 {
                n324 = flat-sequence {
                  tunnel: w421 -> [w424]
                  tunnel: [w424] -> w420
                  tunnel: w419 -> [w423]
                  tunnel: [w422] -> w418
                  tunnel: w420 -> [w428]
                  tunnel: w418 -> [w426]
                  tunnel: w417 -> [w425]
                  frame #0 {
                    n325 = call "CRYSet Graph Cluster Data.vi"("Graph Number"=w423) -> ("DataType"=w422:string)  [unwired: 2 in, 8 out]
                  }
                  frame #1 {
                    n326 = local read "Graph Number"() -> (w427:i32)
                    n327 = Format Into String(w428, w426, w427, 0 ("input 3")) -> (resulting string=w430:string)  [unwired: 3 in, 1 out]
                    n328 = Enqueue Element(queue=w425, element=w430) -> ()  [unwired: 1 in, 4 out]
                  }
                }
              }
            }
          }
          frame "DA_INT_VIEW" {
            n329 = local read "Test"() -> (w432:string)
            n330 = case shown="Default" w432 {
              tunnel: w431 -> [_ w433]
              frame "Test" {
              }
              frame Default {
                n331 = Obtain Queue(name (unnamed)="CURVE" ("YAxisTitle"), element data type="" ("Action Type")) -> (queue out=w440:refnum<queue>)  [unwired: 3 in, 2 out]
                n332 = local read "Graph Number"() -> (w434:i32)
                n333 = Format Into String("Intensity_Insert" ("input 1"), w433, w434, 0 ("input 2")) -> (resulting string=w436:string)  [unwired: 3 in, 1 out]
                n334 = Enqueue Element(queue=w440, element=w436) -> ()  [unwired: 1 in, 4 out]
              }
            }
          }
          frame "DA_PAL_HIDE", "DA_PAL_VIEW" {
            n335 = Equal?(x=w442, y="DA_PAL_VIEW") -> (x = y?=w441:bool)
            n336 = property on="PaletteShow" class="Bool (strict)"("Val(Sgnl)"=w441) -> ()  [unwired: 2 in, 2 out]
          }
          frame "DA_REMOVEALL" {
            n337 = property on="RemoveAll" class="Bool (strict)"("Val(Sgnl)"=TRUE ("Value (Signaling)")) -> ()  [unwired: 2 in, 2 out]
          }
        }
      }
      event Shortcut Menu Activation? {
        n338 = event-data() -> ("MenuRef"=w447:refnum<k9>, "Coords"=w448:T1)  [unwired: 6 out]
        n339 = local read "LegendShow"() -> (w445:bool)
        n340 = case shown="True" w445 {
          selector: w445 -> [_ w453]
          tunnel: w448 -> [_ w464]
          tunnel: w447 -> [_ w462]
          tunnel: w446 -> [_ w458]
          frame False {
          }
          frame True {
            n341 = invoke on="Legend" class="MCListbox (strict)" method="Point To Row Column"("Point"=w464) -> ("CellPosition"=w465:T5)  [unwired: 6 in, 6 out]
            n342 = local read "TotalPlot"() -> (w456:u32)
            n343 = control-ref of="Legend"() -> (w450:refnum<vi>)
            n344 = Unbundle By Name(w465) -> ("Row"=w452:i32)
            n345 = To Long Integer(number=w456) -> (32bit integer=w455:i32)
            n346 = Less?(x=w452, y=w455) -> (x < y?=w460:bool)
            n347 = local write "OldRow"(w452) -> ()
            n348 = Greater?(x=w456, y=u32 0) -> (0:w459:bool)
            n349 = local read "LegendVScrollShow"() -> (w449:bool)
            n350 = call "CRYGet Selected Data in Legend.vi"("Right Clicked Row"=w452, "Legend Ref"=w450) -> ("Selected Rows"=w451:i32[])  [unwired: 9 in]
            n351 = local write "SelectedRow"(w451) -> ()
            n352 = property on="Legend" class="MCListbox (strict)"("Value"=w451) -> ()  [unwired: 2 in, 2 out]
            n353 = Bundle By Name(cluster=w458, "LegendShow"=w453, "CellClick"=w460, "Total Number"=w459, "LegendVScrollShow"=w449) -> (w457:T2)
            n354 = control-ref of="This VI"() -> (w454:refnum<vi>)
            n355 = call "CRYGraph Window Menu.vi"("pGraph VI"=w454, "Flag Cluster"=w457, "Type"="LEGEND", "Runtime Menu Ref In"=w462) -> ()  [unwired: 1 in, 7 out]
          }
        }
        n356 = event-data() -> ()  [unwired: 1 in, 2 out]
      }
      event Shortcut Menu Selection (User) {
        n357 = event-data() -> ("ItemTag"=w469:string)  [unwired: 8 out]
        n358 = local read "Graph Number"() -> (w466:i32)
        n359 = case shown="\"DA_LEG_VSCROLL_HIDE\", \"DA_LEG_VSCROLL_VIEW\"" w469 {
          selector: w469 -> [_ _ _ _ _ _ w503]
          tunnel: w468 -> [_ w474 _ _ _ _ _]
          tunnel: w466 -> [_ w473 _ _ _ _ _]
          frame "", Default {
          }
          frame "DA_LEG_HIDE_1" {
            n360 = Format Into String("DA_LEG_HIDE" ("input 2"), "AAA" ("input 2"), w473, 0 ("input 3")) -> (resulting string=w475:string)  [unwired: 3 in, 1 out]
            n361 = Enqueue Element(queue=w474, element=w475) -> ()  [unwired: 1 in, 4 out]
          }
          frame "DA_LEG_REMOVE" {
            n362 = property on="RemoveSome" class="Bool (strict)"("Val(Sgnl)"=TRUE ("Value (Signaling)")) -> ()  [unwired: 2 in, 2 out]
          }
          frame "DA_LEG_REMOVEALL" {
            n363 = property on="RemoveAll" class="Bool (strict)"("Val(Sgnl)"=TRUE ("Value (Signaling)")) -> ()  [unwired: 2 in, 2 out]
          }
          frame "DA_LEG_INVERT" {
            n364 = local read "TotalPlot"() -> (w479:u32)
            n365 = for {
              N: w479 -> [_]
              tunnel: [w483] -> w480
              tunnel: [w482] -> w478
              i -> [w485]
              w487 = 38
              w489 = 37
              n366 = property on="Legend" class="MCListbox (strict)"() -> ("ItemSyms"=w491:i32[])  [unwired: 2 in, 2 out]
              n367 = Index Array(array=w491, index=w485) -> (element=w490:i32)
              n368 = To Unsigned Long Integer(number=w485) -> (unsigned 32bit integer=w484:u32)
              n369 = Equal?(x=w490, y=w489) -> (x = y?=w486:bool)
              n370 = Equal?(x=w490, y=w487) -> (x = y?=w488:bool)
              n371 = Select(t=w489, s=w488, f=w487) -> (s? t:f=w492:i32)
              n372 = Replace Array Subset(array=w491, new element=w492, index=w485) -> (w493:i32[])
              n373 = property on="WaveGraph" class="WFGraph (strict)"("Active Plot"=w484, "Plot.Visible?"=w486) -> (error out=w482:errorcluster)  [unwired: 2 in, 1 out]
              n374 = property on="Legend" class="MCListbox (strict)"("ItemSyms"=w493) -> (error out=w483:errorcluster)  [unwired: 2 in, 1 out]
            }
            n375 = case shown="No Error" w478 {
              frame No Error {
              }
              frame Error {
              }
            }
            n376 = property on="AxisChange" class="Bool (strict)"(error in=w480, "Val(Sgnl)"=TRUE ("Value (Signaling)")) -> ()  [unwired: 1 in, 2 out]
          }
          frame "DA_LEG_SHOWALL" {
            n377 = local read "TotalPlot"() -> (w494:u32)
            n378 = for {
              N: w494 -> [_]
              tunnel: [38] -> w497 mode=indexing
              i -> [w501]
              n379 = To Unsigned Long Integer(number=w501) -> (unsigned 32bit integer=w500:u32)
              n380 = property on="WaveGraph" class="WFGraph (strict)"("Active Plot"=w500, "Plot.Visible?"=TRUE ("Plot.Visible")) -> ()  [unwired: 2 in, 2 out]
            }
            n381 = property on="Legend" class="MCListbox (strict)"("ItemSyms"=w497) -> (error out=w496:errorcluster)  [unwired: 2 in, 1 out]
            n382 = property on="AxisChange" class="Bool (strict)"(error in=w496, "Val(Sgnl)"=TRUE ("Value (Signaling)")) -> ()  [unwired: 1 in, 2 out]
          }
          frame "DA_LEG_VSCROLL_HIDE", "DA_LEG_VSCROLL_VIEW" {
            n383 = Equal?(x="DA_LEG_VSCROLL_VIEW" ("y"), y=w503) -> (x = y?=w502:bool)
            n384 = property on="LegendVScrollShow" class="Bool (strict)"("Val(Sgnl)"=w502) -> ()  [unwired: 2 in, 2 out]
          }
        }
        n385 = call "CRYPreUpdate Sequence.vi"("EventName"="CurLibUpdate") -> ()  [unwired: 15 in]
      }
      event Shortcut Menu Activation? {
        n386 = event-data() -> ("MenuRef"=w507:refnum<k9>)  [unwired: 7 out]
        n387 = local read "CursorShow"() -> (w505:bool)
        n388 = case shown="True" w505 {
          selector: w505 -> [_ w508]
          tunnel: w507 -> [_ w511]
          tunnel: w506 -> [_ w510]
          frame False {
          }
          frame True {
            n389 = Bundle By Name(cluster=w510, "CursorShow"=w508) -> (w512:T2)
            n390 = control-ref of="This VI"() -> (w509:refnum<vi>)
            n391 = call "CRYGraph Window Menu.vi"("pGraph VI"=w509, "Flag Cluster"=w512, "Type"="CURSOR", "Runtime Menu Ref In"=w511) -> ()  [unwired: 1 in, 7 out]
          }
        }
        n392 = event-data() -> ()  [unwired: 2 in, 1 out]
      }
      event Shortcut Menu Selection (User) {
        n393 = event-data() -> ("ItemTag"=w516:string)  [unwired: 8 out]
        n394 = local read "Graph Number"() -> (w518:i32)
        n395 = Match Pattern(string=w516, regular expression="#" ("search string/char (-)")) -> (before substring=w515:string, after substring=w514:string)  [unwired: 1 in, 2 out]
        n396 = case shown="\"LINKTO\"" w515 {
          selector: w515 -> [_ _ _ w553 _]
          tunnel: w521 -> [_ _ _ w551 w558]
          tunnel: w518 -> [_ _ _ w554 w560]
          tunnel: w520 -> [_ _ _ w552 w559]
          tunnel: w514 -> [w522 _ w537 _ _]
          frame "DA_CUR_GOTO_CUR" {
            n397 = Decimal String To Number(string=w522) -> (number=w523:i32)  [unwired: 1 in, 2 out]
            n398 = case shown="0, 1" w523 {
              selector: w523 -> [_ w525]
              frame Default {
              }
              frame 0, 1 {
                n399 = flat-sequence {
                  tunnel: w525 -> [w527]
                  frame #0 {
                    n400 = Equal To 0?(x=w527) -> (x = 0?=w531:bool)
                    n401 = local write "NewCursIdx"(w527) -> ()
                    n402 = property on="WaveGraph" class="WFGraph (strict)"("Active Cursor"=w527) -> ()  [unwired: 2 in, 2 out]
                    n403 = Select(t=1 ("OldCursIdx"), s=w531, f=0 ("OldCursIdx")) -> (s? t:f=w528:i32)
                    n404 = local write "OldCursIdx"(w528) -> ()
                  }
                  frame #1 {
                    n405 = property on="CursorColor" class="Bool (strict)"("Val(Sgnl)"=TRUE ("Value (Signaling)")) -> ()  [unwired: 2 in, 2 out]
                  }
                }
                n406 = control-ref of="WaveGraph"() -> (w524:refnum<vi>)
                n407 = call "CRYGoto Cursor.vi"("Active Cursor"=w525, "Graph Ref"=w524, "Graph Type"="WAVE") -> ()  [unwired: 9 in]
              }
            }
          }
          frame "DA_BRING_CENTER" {
            n408 = property on="WaveGraph" class="WFGraph (strict)"() -> ("Active Cursor"=w533:u32)  [unwired: 2 in, 2 out]
            n409 = control-ref of="WaveGraph"() -> (w535:refnum<vi>)
            n410 = call "CRYGoto Cursor.vi"("sOption"="Bring_to_Center", "Active Cursor"=w533, "Graph Ref"=w535, "Graph Type"="WAVE") -> ()  [unwired: 8 in]
          }
          frame "LINKTO" {
            n411 = Match Pattern(string=w537, regular expression="[0-1]_") -> (match substring=w541:string, after substring=w539:string)  [unwired: 1 in, 2 out]
            n412 = Decimal String To Number(string=w541) -> (number=w538:i32)  [unwired: 2 in, 1 out]
            n413 = case shown="0, 1" w538 {
              selector: w538 -> [w542 _]
              tunnel: w539 -> [w543 _]
              frame 0, 1 {
                n414 = control-ref of="Legend"() -> (w546:refnum<vi>)
                n415 = local read "Cursor Waves"() -> (w545:string[])
                n416 = call "CRYGet Legend Name.vi"("MCListbox Refnum"=w546) -> ("Names Out"=w547:string[])  [unwired: 10 in]
                n417 = Search 1D Array(1D array=w547, element=w543) -> (index of element=w548:i32)  [unwired: 1 in]
                n418 = Replace Array Subset(array=w545, new element=w543, index=w542) -> (w544:string[])
                n419 = case shown="0, Default" w548 {
                  selector: w548 -> [w549 _]
                  tunnel: w542 -> [w550 _]
                  frame 0, Default {
                    n420 = property on="WaveGraph" class="WFGraph (strict)"("Active Cursor"=w550, "Cursor.Cursor Plot"=w549) -> ()  [unwired: 2 in, 2 out]
                  }
                  frame -1 {
                  }
                }
                n421 = local write "Cursor Waves"(w544) -> ()
              }
              frame Default {
              }
            }
          }
          frame Default {
            n422 = Format Into String(w553, w552, w554, 0 ("input 3")) -> (resulting string=w555:string)  [unwired: 3 in, 1 out]
            n423 = Enqueue Element(queue=w551, element=w555) -> ()  [unwired: 1 in, 4 out]
          }
          frame "DA_CUR_HIDE_1" {
            n424 = Format Into String("DA_CUR_HIDE" ("input 1"), w559, w560, 0 ("input 3")) -> (resulting string=w561:string)  [unwired: 3 in, 1 out]
            n425 = Enqueue Element(queue=w558, element=w561) -> ()  [unwired: 1 in, 4 out]
          }
        }
        n426 = call "CRYPreUpdate Sequence.vi"("EventName"="CurLibUpdate") -> ()  [unwired: 15 in]
      }
      event Shortcut Menu Activation? {
        n427 = event-data() -> ("MenuRef"=w564:refnum<k9>)  [unwired: 7 out]
        n428 = local read "PreviewShow"() -> (w563:bool)
        n429 = case shown="True" w563 {
          selector: w563 -> [_ w566]
          tunnel: w565 -> [_ w568]
          tunnel: w564 -> [_ w567]
          frame False {
          }
          frame True {
            n430 = Bundle By Name(cluster=w568, "PreviewShow"=w566) -> (w570:T2)
            n431 = control-ref of="This VI"() -> (w569:refnum<vi>)
            n432 = call "CRYGraph Window Menu.vi"("pGraph VI"=w569, "Flag Cluster"=w570, "Type"="PREVIEW", "Runtime Menu Ref In"=w567) -> ()  [unwired: 1 in, 7 out]
          }
        }
        n433 = event-data() -> ()  [unwired: 2 in, 1 out]
      }
      event Shortcut Menu Selection (User) {
        n434 = event-data() -> ("ItemTag"=w573:string)  [unwired: 8 out]
        n435 = case shown="\"DA_PRE_LOCATION\"" w573 {
          tunnel: w572 -> [_ _ _ w642]
          frame Default {
          }
          frame "DA_PRE_SHOWALL" {
            n436 = flat-sequence {
              frame #0 {
                n437 = property on="WaveGraph" class="WFGraph (strict)"("ActXScl"=0 ("Active X Scale"), "XScale.ScaleFit"=u8 2 ("X Scale.Scale Fit")) -> ()  [unwired: 2 in, 2 out]
                n438 = property on="PreviewGraph" class="WFGraph (strict)"() -> ("XScale.Maximum"=w576:dbl, "XScale.Minimum"=w575:dbl)  [unwired: 2 in, 2 out]
                n439 = property on="WaveGraph" class="WFGraph (strict)"("XScale.Maximum"=w576, "XScale.Minimum"=w575) -> ()  [unwired: 2 in, 2 out]
              }
              frame #1 {
                n440 = property on="ScaleRange" class="Bool (strict)"("Val(Sgnl)"=TRUE ("Value (Signaling)")) -> ()  [unwired: 2 in, 2 out]
              }
            }
          }
          frame "DA_PRE_LOCATION" {
            n441 = flat-sequence {
              frame #0 {
                n442 = property on="Scrollbar" class="Scroll (strict)"() -> ("PageSize"=w583:dbl, "Value"=w582:dbl)  [unwired: 2 in, 2 out]
                n443 = local read "PreviewCoords"() -> (w602:T1)
                n444 = property on="PreviewGraph" class="WFGraph (strict)"() -> ("Plot Bounds"=w606:T6, "Width"=w605:u32)  [unwired: 2 in, 2 out]
                n445 = Equal?(x=w583, y=w582) -> (x = y?=w581:bool)
                n446 = property on="WaveGraph" class="WFGraph (strict)"("XScale.ScaleFit"=u8 0 ("X Scale.Scale Fit"), "ActYScl"=0 ("Active Y Scale")) -> ()  [unwired: 2 in, 2 out]
                n447 = case shown="True" w581 {
                  tunnel: [w614 w619] -> w601
                  frame False {
                    n448 = property on="PreviewGraph" class="WFGraph (strict)"("Active Cursor"=u32 0, "Active Cursor"=u32 1) -> ("Cursor.Cursor X"=w612:dbl, "Cursor.Cursor X"=w613:dbl)  [unwired: 2 in, 2 out]
                    n449 = Greater?(x=w612, y=w613) -> (0:w611:bool)
                    n450 = case shown="True" w611 {
                      tunnel: w612 -> [w616 w618]
                      tunnel: w613 -> [w615 w617]
                      tunnel: [w616 w617] -> w607
                      tunnel: [w615 w618] -> w608
                      frame False {
                      }
                      frame True {
                      }
                    }
                    n451 = Subtract(x=w608, y=w607) -> (x-y=w614:dbl)
                  }
                  frame True {
                    n452 = property on="PreviewGraph" class="WFGraph (strict)"("ActXScl"=0 ("Active X Scale")) -> ("XScale.Maximum"=w623:dbl, "XScale.Minimum"=w622:dbl)  [unwired: 2 in, 2 out]
                    n453 = Subtract(x=w623, y=w622) -> (x-y=w621:dbl)
                    n454 = Divide(x=w621, y=20.0) -> (x/y=w619:dbl)
                  }
                }
                n455 = Unbundle By Name(w602) -> ("Horizontal"=w595:i32)
                n456 = To Long Integer(number=w605) -> (32bit integer=w590:i32)
                n457 = Unbundle By Name(w606) -> ("Left"=w604:i16)
                n458 = To Long Integer(number=w604) -> (32bit integer=w593:i32)
                n459 = Add(x=w593, y=w590) -> (x+y=w603:i32)
                n460 = Less?(x=w595, y=w593) -> (x < y?=w599:bool)
                n461 = Greater?(x=w595, y=w603) -> (0:w598:bool)
                n462 = property on="PreviewGraph" class="WFGraph (strict)"("ActXScl"=0 ("Active X Scale")) -> ("XScale.Maximum"=w586:dbl, "XScale.Minimum"=w588:dbl)  [unwired: 2 in, 2 out]
                n463 = Build Array(w599, w598) -> (w597:bool[])
                n464 = Search 1D Array(1D array=w597, element=TRUE) -> (index of element=w592:i32)  [unwired: 1 in]
                n465 = Divide(x=w601, y=2.0) -> (x/y=w594:dbl)
                n466 = Subtract(x=w586, y=w588) -> (x-y=w589:dbl)
                n467 = case shown="0" w592 {
                  tunnel: w595 -> [_ _ w639]
                  tunnel: [w625 w629 w631] -> w587
                  tunnel: w594 -> [w627 w630 _]
                  tunnel: w593 -> [_ _ w638]
                  tunnel: w590 -> [_ _ w636]
                  tunnel: w589 -> [_ _ w634]
                  tunnel: w588 -> [w626 _ w632]
                  tunnel: w586 -> [_ w628 _]
                  frame 0 {
                    n468 = Add(x=w627, y=w626) -> (x+y=w625:dbl)
                  }
                  frame 1 {
                    n469 = Subtract(x=w628, y=w630) -> (x-y=w629:dbl)
                  }
                  frame Default {
                    n470 = Subtract(x=w639, y=w638) -> (x-y=w637:i32)
                    n471 = Divide(x=w637, y=w636) -> (x/y=w635:dbl)
                    n472 = Multiply(x=w635, y=w634) -> (x*y=w633:dbl)
                    n473 = Add(x=w633, y=w632) -> (x+y=w631:dbl)
                  }
                }
                n474 = Add(x=w587, y=w594) -> (x+y=w585:dbl)
                n475 = Subtract(x=w587, y=w594) -> (x-y=w584:dbl)
                n476 = property on="WaveGraph" class="WFGraph (strict)"("XScale.Maximum"=w585, "XScale.Minimum"=w584) -> ()  [unwired: 2 in, 2 out]
              }
              frame #1 {
                n477 = property on="ScaleRange" class="Bool (strict)"("Val(Sgnl)"=TRUE ("Value (Signaling)")) -> ()  [unwired: 2 in, 2 out]
              }
            }
          }
          frame "DA_PRE_HIDE_1" {
            n478 = local read "Graph Number"() -> (w641:i32)
            n479 = Format Into String("DA_PRE_HIDE" ("input 2"), "AAA" ("input 2"), w641, 0 ("input 3")) -> (resulting string=w646:string)  [unwired: 3 in, 1 out]
            n480 = Enqueue Element(queue=w642, element=w646) -> ()  [unwired: 1 in, 4 out]
          }
        }
      }
      event "PaletteShow": Value Change {
        n481 = event-data() -> ("NewVal"=w647:bool)  [unwired: 6 out]
        n482 = property on="WaveGraph" class="WFGraph (strict)"("Palette Visible"=w647) -> ()  [unwired: 2 in, 2 out]
      }
      event "Cursor": Key Down {
        n483 = event-data() -> ("ScanCode"=w648:i16)  [unwired: 10 out]
        n484 = case shown="75, 77" w648 {
          selector: w648 -> [_ w651]
          tunnel: w649 -> [_ w652]
          frame Default {
          }
          frame 75, 77 {
            n485 = flat-sequence {
              tunnel: w651 -> [w655]
              tunnel: [w655] -> w650
              tunnel: w652 -> [w664]
              tunnel: w650 -> [w661]
              frame #0 {
                n486 = local write "CursorMoveFinish"(TRUE ("CursorMove")) -> ()
                n487 = local write "KeyRepeatCount"(1 ("KeyRepeatCount")) -> ()
              }
              frame #1 {
                n488 = Equal?(x=i16 75, y=w661) -> (x = y?=w657:bool)
                n489 = Select(t="Left" ("input 2"), s=w657, f="Right" ("input 2")) -> (s? t:f=w656:string)
                n490 = To Long Integer(number=w661) -> (32bit integer=w663:i32)
                n491 = local write "WhichKey"(w656) -> ()
                n492 = Format Into String("Cursor_Move" ("input 1"), w656, w663, 0 ("input 4")) -> (resulting string=w665:string)  [unwired: 3 in, 1 out]
                n493 = Enqueue Element(queue=w664, element=w665) -> ()  [unwired: 1 in, 4 out]
              }
            }
          }
        }
      }
      event "Cursor": Key Repeat {
        n494 = event-data() -> ("ScanCode"=w667:i16)  [unwired: 10 out]
        n495 = case shown="75, 77" w667 {
          selector: w667 -> [_ w670]
          tunnel: w668 -> [_ w671]
          frame Default {
          }
          frame 75, 77 {
            n496 = flat-sequence {
              tunnel: w670 -> [w674]
              tunnel: [w674] -> w669
              tunnel: w671 -> [w679]
              tunnel: w669 -> [w677]
              frame #0 {
                n497 = local read "KeyRepeatCount"() -> (w673:i32)
                n498 = Increment(x=w673) -> (x+1=w672:i32)
                n499 = local write "KeyRepeatCount"(w672) -> ()
              }
              frame #1 {
                n500 = local read "WhichKey"() -> (w675:string)
                n501 = To Long Integer(number=w677) -> (32bit integer=w678:i32)
                n502 = Format Into String("Cursor_Move" ("input 1"), w675, w678, 0 ("input 4")) -> (resulting string=w680:string)  [unwired: 3 in, 1 out]
                n503 = Enqueue Element(queue=w679, element=w680) -> ()  [unwired: 1 in, 4 out]
              }
            }
          }
        }
      }
      event "Cursor": Key Up {
        n504 = event-data() -> ("ScanCode"=w682:i16)  [unwired: 7 out]
        n505 = case shown="75, 77" w682 {
          selector: w682 -> [_ w685]
          tunnel: w683 -> [_ w686]
          frame Default {
          }
          frame 75, 77 {
            n506 = flat-sequence {
              tunnel: w685 -> [w688]
              tunnel: [w688] -> w684
              tunnel: w686 -> [w697]
              tunnel: w684 -> [w693]
              frame #0 {
                n507 = local write "CursorMoveFinish"(FALSE ("CursorMoveFinish")) -> ()
              }
              frame #1 {
                n508 = Equal?(x=i16 75, y=w693) -> (x = y?=w692:bool)
                n509 = Select(t="Left" ("input 2"), s=w692, f="Right" ("input 2")) -> (s? t:f=w689:string)
                n510 = To Long Integer(number=w693) -> (32bit integer=w696:i32)
                n511 = local write "WhichKey"(w689) -> ()
                n512 = Format Into String("Cursor_Move" ("input 1"), w689, w696, 0 ("input 4")) -> (resulting string=w698:string)  [unwired: 3 in, 1 out]
                n513 = Enqueue Element(queue=w697, element=w698) -> ()  [unwired: 1 in, 4 out]
              }
            }
          }
        }
      }
      event "Cursor": Mouse Down {
        n514 = event-data() -> ("CtlRef"=w703:refnum<vi>, "Coords"=w700:T1)  [unwired: 7 out]
        n515 = invoke class="Tbl (strict)" method="Point To Row Column"(reference=w703, "Point"=w700) -> ("CellPosition"=w702:T5)  [unwired: 4 in, 5 out]
        n516 = local write "Cursor Coords"(w700) -> ()
        n517 = Unbundle By Name(w702) -> ("Row"=w701:i32)
        n518 = flat-sequence {
          tunnel: w701 -> [w704]
          frame #0 {
            n519 = Equal To 0?(x=w704) -> (x = 0?=w708:bool)
            n520 = local write "NewCursIdx"(w704) -> ()
            n521 = property on="WaveGraph" class="WFGraph (strict)"("Active Cursor"=w704) -> ()  [unwired: 2 in, 2 out]
            n522 = Select(t=1 ("OldCursIdx"), s=w708, f=0 ("OldCursIdx")) -> (s? t:f=w705:i32)
            n523 = local write "OldCursIdx"(w705) -> ()
          }
          frame #1 {
            n524 = property on="CursorColor" class="Bool (strict)"("Val(Sgnl)"=TRUE ("Value (Signaling)")) -> ()  [unwired: 2 in, 2 out]
          }
        }
      }
      event "Cursor": Value Change {
        n525 = event-data() -> ("OldVal"=w714:string[][], "NewVal"=w713:string[][])  [unwired: 5 out]
        n526 = local read "Cursor Coords"() -> (w711:T1)
        n527 = control-ref of="This VI"() -> (w712:refnum<vi>)
        n528 = call "CRYCursor move in Cursor Table.vi"("NewVal"=w713, "OldVal"=w714, "Cursor Coords"=w711, "pGraph VI"=w712) -> ("NewVal Out"=w710:string[][])  [unwired: 7 in]
        n529 = local write "Cursor"(w710) -> ()
      }
      event "CursorShow": Value Change {
        n530 = event-data() -> ("NewVal"=w715:bool)  [unwired: 6 out]
        n531 = flat-sequence {
          tunnel: w715 -> [w720]
          frame #0 {
            n532 = Select(t="DA_CUR_VIEW", s=w720, f="DA_CUR_HIDE") -> (s? t:f=w719:string)
            n533 = control-ref of="This VI"() -> (w716:refnum<vi>)
            n534 = call "CRYCursor InsDel.vi"("Graph VI Ref"=w716, "sAction"=w719) -> ()  [unwired: 10 in]
          }
          frame #1 {
            n535 = property on="ToolbarUpdate" class="Bool (strict)"("Val(Sgnl)"=TRUE ("Value (Signaling)")) -> ()  [unwired: 2 in, 2 out]
          }
        }
      }
      event "CursorPlot": Value Change {
        # "for cursor moving by keydown"
        n536 = event-data() -> ()  [unwired: 7 out]
        n537 = local read "CursorShow"() -> (w722:bool)
        n538 = case shown="True" w722 {
          frame False {
          }
          frame True {
            n539 = control-ref of="WaveGraph"() -> (w725:refnum<vi>)
            n540 = control-ref of="Cursor"() -> (w724:refnum<vi>)
            n541 = call "CRYPlot Cursor.vi"("Cursor Ref"=w724, "Graph Ref"=w725, "Graph Type"="WAVE") -> ()  [unwired: 9 in]
          }
        }
      }
      event "CursorColor": Value Change {
        n542 = event-data() -> ()  [unwired: 7 out]
        n543 = local read "NewCursIdx"() -> (w736:u32)
        n544 = local read "OldCursIdx"() -> (w737:u32)
        n545 = property on="WaveGraph" class="WFGraph (strict)"("Active Cursor"=w737) -> ("Cursor.Cursor Color"=w729:u32)  [unwired: 2 in, 2 out]
        n546 = property on="WaveGraph" class="WFGraph (strict)"("Active Cursor"=w736) -> ("Cursor.Cursor Color"=w728:u32)  [unwired: 2 in, 2 out]
        n547 = Bundle By Name(cluster=T5 {"Row"=0, "Column"=0} ("Active Cell:Active Cell"), "Row"=w736, "Column"=0) -> (w733:T5)
        n548 = Bundle By Name(cluster=T5 {"Row"=0, "Column"=0} ("Active Cell:Active Cell"), "Row"=w737, "Column"=0) -> (w730:T5)
        n549 = property on="Cursor" class="Tbl (strict)"("Active Cell"=w730, "CellFontColor"=w729, "Cell BG Color"=u32 16777226) -> ()  [unwired: 2 in, 2 out]
        n550 = property on="Cursor" class="Tbl (strict)"("Active Cell"=w733, "CellFontColor"=w728, "Cell BG Color"=u32 60927) -> ()  [unwired: 2 in, 2 out]
      }
      event "Legend": Mouse Down {
        n551 = event-data() -> ("CtlRef"=w739:refnum<vi>, "Coords"=w744:T1, "Button"=w743:u16)  [unwired: 6 out]
        n552 = local read "TotalPlot"() -> (w740:u32)
        n553 = call "CRYData View Legend Plot OnOff.vi"("TotalPlot"=w740, "Button Info"=w743, "Mouse Point"=w744, "MCListbox Ref In"=w739) -> ("Active Row"=w738:i32, "Visible?"=w741:bool, "Click State"=w742:bool)  [unwired: 5 out]
        n554 = case shown="True" w742 {
          tunnel: w741 -> [_ w750]
          tunnel: w738 -> [_ w751]
          frame False {
          }
          frame True {
            n555 = property on="WaveGraph" class="WFGraph (strict)"("XScale.ScaleFit"=u8 0 ("Y Scale.Scale Fit")) -> (error out=w747:errorcluster)  [unwired: 2 in, 1 out]
            n556 = property on="AxisChange" class="Bool (strict)"("Val(Sgnl)"=TRUE ("Value (Signaling)")) -> ()  [unwired: 2 in, 2 out]
            n557 = To Unsigned Long Integer(number=w751) -> (unsigned 32bit integer=w749:u32)
            n558 = property on="WaveGraph" class="WFGraph (strict)"(error in=w747, "Active Plot"=w749, "Plot.Visible?"=w750) -> (error out=w745:errorcluster)  [unwired: 1 in, 1 out]
            n559 = case shown="No Error" w745 {
              frame No Error {
              }
              frame Error {
              }
            }
          }
        }
      }
      event "Legend": Double Click {
        n560 = event-data() -> ("CtlRef"=w753:refnum<vi>, "Coords"=w752:T1)  [unwired: 8 out]
        n561 = disable-structure shown="Disabled" {
          disable-tunnel: w753 -> [w759 _]
          disable-tunnel: w752 -> [w758 _]
          frame Disabled {
            n562 = call "CRYGet MultiListBox Click State.vi"("Coords"=w758, "MultiList Box Ref In"=w759) -> ("State"=w757:bool)  [unwired: 6 in, 3 out]
            n563 = call "CRYClick Name in Legend.vi"("Mouse Point"=w758, "MCListbox Ref In"=w759) -> ("Active Row"=w755:i32, "Click State?"=w756:bool)  [unwired: 8 in]
            n564 = And(x=w757, y=w756) -> (x .and. y?=w754:bool)
            n565 = case shown="True" w754 {
              tunnel: w759 -> [_ w760]
              tunnel: w755 -> [_ w761]
              frame False {
              }
              frame True {
                n566 = call "CRYOpen Step by Legend.vi"("Active Row"=w761, "MCListbox Ref In"=w760, "Type"=enum16{"Curves", "Values", "Results", "WFM"}."WFM" ("Type In")) -> ()  [unwired: 9 in]
              }
            }
          }
          frame Enabled {
          }
        }
      }
      event "Legend": Mouse Move {
        n567 = event-data() -> ("Coords"=w770:T1)  [unwired: 5 out]
        n568 = control-ref of="Legend"() -> (w763:refnum<vi>)
        n569 = local read "TotalPlot"() -> (w769:u32)
        n570 = call "CRYData View Legend Mouse Move.vi"("TotalPlot"=w769, "Mouse Point"=w770, "MCListbox Ref In"=w763) -> ("CellSize"=w767:T7, "Position"=w766:T8, "Selected Row"=w765:i32, "Move State"=w764:bool, "CellBG"=w768:u32)  [unwired: 1 in, 3 out]
        n571 = case shown="True" w764 {
          tunnel: w768 -> [_ w776]
          tunnel: w767 -> [_ w775]
          tunnel: w766 -> [_ w774]
          tunnel: w765 -> [_ w773]
          frame False {
            n572 = property on="ColorBox" class="ColBox"("Visible"=FALSE) -> ()  [unwired: 2 in, 2 out]
          }
          frame True {
            n573 = local write "OldRow"(w773) -> ()
            n574 = property on="ColorBox" class="ColBox"("Position"=w774, "Color Area Size"=w775, "Value"=w776, "Visible"=TRUE) -> ()  [unwired: 2 in, 2 out]
          }
        }
      }
      event "Legend": Value Change {
        n575 = event-data() -> ("NewVal"=w777:i32[])  [unwired: 6 out]
        n576 = local read "Test"() -> (w778:string)
        n577 = case shown="Default" w778 {
          tunnel: w777 -> [_ w780]
          frame "Test" {
          }
          frame Default {
            n578 = local read "GraphType"() -> (w782:string)
            n579 = control-ref of="Legend"() -> (w781:refnum<vi>)
            n580 = call "CRYData View Legend Manipulate.vi"("sAction"="GetViewNumbyLegNum", "nData"=w780, "sData"=w782, "Legend Ref"=w781) -> ("nData Out"=w783:i32[])  [unwired: 6 in, 1 out]
            n581 = call "CRYGet Graph Name From Graph Type.vi"("Graph Type"=w782) -> ("Type"=w785:enum16{"Curves", "Values", "Results", "WFM"})  [unwired: 9 in, 1 out]
            n582 = call "CRYTree Global Manipulate.vi"("Type In"=w785) -> ("Tree/Curve Tree"=w784:refnum<vi>)  [unwired: 7 in, 3 out]
            n583 = call "CRYTree Manuplate.vi"("sAction"="SetActiveNumbers", "nData"=w783, "Tree in"=w784) -> ("Tree Out"=w779:refnum<vi>)  [unwired: 5 in, 3 out]
            n584 = flat-sequence {
              tunnel: w779 -> [_]
              frame #0 {
                n585 = call "CRYUpdate Buttons.vi"() -> ()  [unwired: 12 in]
              }
            }
          }
        }
      }
      event "LegendVScrollShow": Value Change {
        w799 = T6 {"Left"=0, "Top"=0, "Right"=0, "Bottom"=0}  # input cluster
        n586 = event-data() -> ("NewVal"=w789:bool)  [unwired: 6 out]
        n587 = property on="Legend" class="MCListbox (strict)"("VScrollVis"=w789) -> ()  [unwired: 2 in, 2 out]
        n588 = control-ref of="PaneLegend"() -> (w791:refnum<vi>)
        n589 = property class="Pane"(reference=w791) -> ("Left"=w798:i32, "Top"=w795:i32, "Width"=w797:u32, "Height"=w794:u32)  [unwired: 1 in, 2 out]
        n590 = Add(x=w798, y=w797) -> (x+y=w796:u32)
        n591 = Add(x=w795, y=w794) -> (x+y=w793:u32)
        n592 = Bundle By Name(cluster=w799, "Left"=w798, "Top"=w795, "Right"=w796, "Bottom"=w793) -> (w792:T6)
        n593 = control-ref of="Legend"() -> (w790:refnum<vi>)
        n594 = local read "LegendVScrollShow"() -> (w788:bool)
        n595 = call "CRYLegend Resize in Graph Window.vi"("VScrollShow"=w788, "Pane Ref"=w791, "input cluster"=w792, "Legend"=w790) -> ()  [unwired: 8 out]
      }
      event "RemoveAll": Value Change {
        w805 = 0 ("Active X Scale")
        w803 = "" ("X Scale.Name Label.Text")
        n596 = event-data() -> ()  [unwired: 7 out]
        n597 = flat-sequence {
          frame #0 {
            n598 = control-ref of="This VI"() -> (w829:refnum<vi>)
            n599 = Build Array(-1 ("nData")) -> (w830:i32[])
            n600 = call "CRYSymbol Conversion.vi"("pGraph VI"=w829, "CurLib Tab Type"=enum16{"Curves", "Values", "Results", "WFM"}."WFM", "nDatas"=w830, "sActin"="LEGEND_REMOVE") -> ()  [unwired: 8 in]
          }
          frame #1 {
            n601 = control-ref of="Legend"() -> (w833:refnum<vi>)
            n602 = call "CRYData View Legend Item Delete.vi"("RowNumber"=-1, "Legend MultiListbox In"=w833) -> ()  [unwired: 10 out]
          }
        }
        n603 = local write "TotalPlot"(u32 0 ("TotalPlot")) -> ()
        n604 = local write "OldRow"(-1 ("OldRow 2")) -> ()
        n605 = flat-sequence {
          tunnel: w801 -> [w811]
          tunnel: [w811] -> w800
          tunnel: w800 -> [w819]
          frame #0 {
            n606 = local read "CursorShow"() -> (w812:bool)
            n607 = case shown="True" w812 {
              tunnel: w811 -> [_ w815]
              frame False {
              }
              frame True {
                n608 = local read "Graph Number"() -> (w814:i32)
                n609 = Format Into String("DA_CUR_HIDE" ("input 1"), "AAA" ("input 2"), w814, 0 ("input 3")) -> (resulting string=w817:string)  [unwired: 3 in, 1 out]
                n610 = Enqueue Element(queue=w815, element=w817) -> ()  [unwired: 1 in, 4 out]
              }
            }
          }
          frame #1 {
            n611 = local read "PreviewShow"() -> (w820:bool)
            n612 = case shown="True" w820 {
              tunnel: w819 -> [_ w823]
              frame False {
              }
              frame True {
                n613 = local read "Graph Number"() -> (w822:i32)
                n614 = Format Into String("DA_PRE_HIDE" ("input 1"), "AAA" ("input 2"), w822, 0 ("input 3")) -> (resulting string=w825:string)  [unwired: 3 in, 1 out]
                n615 = Enqueue Element(queue=w823, element=w825) -> ()  [unwired: 1 in, 4 out]
              }
            }
          }
        }
        n616 = local write "CursorEnabled"(FALSE ("CursorEnabled")) -> ()
        n617 = property on="WaveGraph" class="WFGraph (strict)"("ActXScl"=w805, "XScale.NameLbl.Text"=w803, "ActYScl"=w805, "YScale.NameLbl.Text"=w803, "ActYScl"=1 ("Active Y Scale"), "YScale.NameLbl.Text"=w803, "YScale.Visible"=FALSE ("Y Scale.Visible")) -> ()  [unwired: 2 in, 2 out]
        n618 = flat-sequence {
          frame #0 {
            n619 = local write "WaveGraph"(cluster{"xo":dbl, "dx":dbl, dbl[]}[] [{"xo"=0.0, "dx"=0.0, [0.0]}] ("appended array")) -> ()
          }
          frame #1 {
            n620 = property on="Repaint Watermark" class="DigNum (strict)"("Val(Sgnl)"=-1 ("y")) -> ()  [unwired: 2 in, 2 out]
          }
        }
      }
      event "RemoveSome": Value Change {
        n621 = event-data() -> ()  [unwired: 7 out]
        n622 = flat-sequence {
          tunnel: [w837] -> w835
          tunnel: [w845] -> w834
          tunnel: w835 -> [w868]
          tunnel: w834 -> [w867]
          frame #0 {
            n623 = local read "SelectedRow"() -> (w844:i32[])
            n624 = Reverse 1D Array(array=w844) -> (reversed array=w837:i32[])
            n625 = control-ref of="Legend"() -> (w840:refnum<vi>)
            n626 = for {
              shift-right: [w848] -> w845
              shift-left: _ -> [w847]
              tunnel: w837 -> [w846] mode=indexing
              n627 = local read "TotalPlot"() -> (w852:u32)
              n628 = Decrement(x=w852) -> (x-1=w851:u32)
              n629 = Increment(x=w846) -> (x+1=w849:i32)
              n630 = Subtract(x=w851, y=w846) -> (x-y=w850:u32)
              n631 = for {
                N: w850 -> [_]
                tunnel: w849 -> [w859]
                shift-right: [w855] -> w848
                shift-left: w847 -> [w854]
                i -> [w858]
                n632 = Add(x=w859, y=w858) -> (x+y=w856:i32)
                n633 = Decrement(x=w856) -> (x-1=w857:i32)
                n634 = property on="WaveGraph" class="WFGraph (strict)"(error in=w854, "Active Plot"=w856) -> (error out=w853:errorcluster, "Plot.Plot Color"=w866:u32, "Plot.Fill/Pt. Color"=w865:u32, "Plot.Fill To"=w864:i16, "Plot.Line Style"=w863:u8, "Plot.Line Width"=w862:u8, "Plot.Point Style"=w861:u8, "Plot.Plot Interpolation"=w860:u8)  [unwired: 1 in, 1 out]
                n635 = property on="WaveGraph" class="WFGraph (strict)"(error in=w853, "Active Plot"=w857, "Plot.Plot Color"=w866, "Plot.Fill/Pt. Color"=w865, "Plot.Fill To"=w864, "Plot.Line Style"=w863, "Plot.Line Width"=w862, "Plot.Point Style"=w861, "Plot.Plot Interpolation"=w860) -> (error out=w855:errorcluster)  [unwired: 1 in, 1 out]
              }
              n636 = local write "TotalPlot"(w851) -> ()
            }
            n637 = local read "GraphType"() -> (w838:string)
            n638 = call "CRYData View Legend Manipulate.vi"("sAction"="GetGlobalNumbyLegNum", "nData"=w837, "sData"=w838, "Legend Ref"=w840) -> ("nData Out"=w839:i32[])  [unwired: 6 in, 1 out]
            n639 = control-ref of="This VI"() -> (w842:refnum<vi>)
            n640 = call "CRYSymbol Conversion.vi"("pGraph VI"=w842, "CurLib Tab Type"=enum16{"Curves", "Values", "Results", "WFM"}."WFM", "nDatas"=w839, "sActin"="LEGEND_REMOVE") -> ()  [unwired: 8 in]
          }
          frame #1 {
            n641 = case shown="No Error" w867 {
              frame No Error {
              }
              frame Error {
              }
            }
            n642 = for {
              tunnel: w868 -> [w869] mode=indexing
              n643 = local read "WaveGraph"() -> (w871:cluster{"xo":dbl, "dx":dbl, dbl[]}[])
              n644 = control-ref of="Legend"() -> (w872:refnum<vi>)
              n645 = Delete From Array(array=w871, index=w869) -> (array with subset deleted=w870:cluster{"xo":dbl, "dx":dbl, dbl[]}[])  [unwired: 1 in, 1 out]
              n646 = call "CRYData View Legend Item Delete.vi"("RowNumber"=w869, "Legend MultiListbox In"=w872) -> ()  [unwired: 10 out]
              n647 = local write "WaveGraph"(w870) -> ()
            }
          }
          frame #2 {
            n648 = local read "TotalPlot"() -> (w874:u32)
            n649 = case shown="1, Default" w874 {
              selector: w874 -> [_ w878]
              frame 0 {
                n650 = property on="RemoveAll" class="Bool (strict)"("Val(Sgnl)"=TRUE ("Value (Signaling)")) -> ()  [unwired: 2 in, 2 out]
              }
              frame 1, Default {
                n651 = for {
                  N: w878 -> [_]
                  tunnel: [w881] -> w876
                  i -> [w884]
                  n652 = property on="Legend" class="MCListbox (strict)"() -> ("ItemSyms"=w887:i32[])  [unwired: 2 in, 2 out]
                  n653 = Bundle By Name(cluster=T5 {"Row"=0, "Column"=0} ("Active Cell:Active Cell"), "Row"=w884, "Column"=1) -> (w888:T5)
                  n654 = Index Array(array=w887, index=w884) -> (element=w885:i32)
                  n655 = property on="Legend" class="MCListbox (strict)"("ActiveCell"=w888) -> ("CellBG"=w883:u32)  [unwired: 2 in, 2 out]
                  n656 = Equal?(x=w885, y=38) -> (x = y?=w882:bool)
                  n657 = property on="WaveGraph" class="WFGraph (strict)"("Active Plot"=w884, "Plot.Plot Color"=w883, "Plot.Fill/Pt. Color"=w883, "Plot.Visible?"=w882) -> (error out=w881:errorcluster)  [unwired: 2 in, 1 out]
                }
                n658 = local read "PreviewShow"() -> (w877:bool)
                n659 = case shown="True" w877 {
                  frame False {
                  }
                  frame True {
                    n660 = control-ref of="This VI"() -> (w879:refnum<vi>)
                    n661 = call "CRYPlot Wave Graph Preview.vi"("sOption"="Update", "Graph VI Ref"=w879) -> ()  [unwired: 10 in]
                  }
                }
                n662 = case shown="No Error" w876 {
                  frame No Error {
                  }
                  frame Error {
                  }
                }
              }
            }
            n663 = property on="AxisChange" class="Bool (strict)"("Val(Sgnl)"=TRUE ("Value (Signaling)")) -> ()  [unwired: 2 in, 2 out]
          }
        }
      }
      event "AxisChange": Value Change {
        w894 = enum16{"Curves", "Values", "Results", "WFM"}."WFM" ("Type In")
        n664 = event-data() -> ()  [unwired: 7 out]
        n665 = control-ref of="Legend"() -> (w905:refnum<vi>)
        n666 = call "CRYGet Graph Data in Graph.vi"("Graph Type"="WAVE", "Legend Refnum"=w905, "Type In"=w894) -> ("Rows"=w903:i32[])  [unwired: 4 in, 4 out]
        n667 = property on="Legend" class="MCListbox (strict)"() -> ("ItemSyms"=w902:i32[])  [unwired: 2 in, 2 out]
        n668 = for {
          tunnel: w902 -> [w916] mode=indexing
          shift-right: [w915] -> w901
          shift-left: i32[] [] -> [w914]
          tunnel: w903 -> [w913] mode=indexing
          shift-right: [w910] -> w895
          shift-left: i32[] [] -> [w909]
          i -> [w911]
          n669 = Equal?(x=38, y=w916) -> (x = y?=w912:bool)
          n670 = case shown="True" w912 {
            tunnel: [w919 w925] -> w915
            tunnel: w914 -> [w919 w924]
            tunnel: w913 -> [_ w923]
            tunnel: w911 -> [_ w922]
            tunnel: [w918 w921] -> w910
            tunnel: w909 -> [w918 w920]
            frame False {
            }
            frame True {
              n671 = Insert Into Array(array=w920, new element=w922) -> (w921:i32[])  [unwired: 1 in]
              n672 = Insert Into Array(array=w924, new element=w923) -> (w925:i32[])  [unwired: 1 in]
            }
          }
        }
        n673 = call "CRYGet Legend Name.vi"("MCListbox Refnum"=w905) -> ("Names Out"=w899:string[])  [unwired: 10 in]
        n674 = control-ref of="This VI"() -> (w891:refnum<vi>)
        n675 = for {
          tunnel: w899 -> [w931]
          tunnel: w895 -> [w932] mode=indexing
          tunnel: [w929] -> w896 mode=indexing
          tunnel: [w928] -> w898
          tunnel: w894 -> [w927]
          n676 = Index Array(array=w931, index=w932) -> (element=w930:string)
          n677 = call "CRYGet Curve Library Data.vi"("Type"=w927, "Data Name"=w930) -> ("Wave"=w926:T9)  [unwired: 4 out]
          n678 = Unbundle By Name(w926) -> ("Y unit"=w929:string, "X unit"=w928:string)
        }
        n679 = call "CRYGet Two Units Rows.vi"("pGraph VI In"=w891, "Old Rows In"=w901, "Type"=w894) -> ("Unit2"=w907:string, "Unit1"=w897:string, "Two Units"=w908:i32)  [unwired: 2 in, 4 out]
        n680 = for {
          tunnel: w895 -> [w941] mode=indexing
          tunnel: w896 -> [w939] mode=indexing
          tunnel: w897 -> [w940]
          shift-right: [w934] -> w892
          shift-left: _ -> [w933]
          n681 = Equal?(x=w940, y=w939) -> (x = y?=w938:bool)
          n682 = Select(t=u32 0 ("Plot.Y Scale Index"), s=w938, f=u32 1 ("Plot.Y Scale Index")) -> (s? t:f=w935:u32)
          n683 = property on="WaveGraph" class="WFGraph (strict)"(error in=w933, "Active Plot"=w941, "Plot.YScaleIdx"=w935) -> (error out=w934:errorcluster)  [unwired: 1 in, 1 out]
        }
        n684 = case shown="2, Default" w908 {
          tunnel: w897 -> [w945 _ w960]
          tunnel: w907 -> [w947 _ _]
          tunnel: w898 -> [w943 _ w958]
          tunnel: [-1 ("Two Units") -1 ("Two Units") -1 ("Two Units")] -> w893
          frame 2, Default {
            n685 = property on="WaveGraph" class="WFGraph (strict)"("ActXScl"=0 ("Active X Scale"), "XScale.NameLbl.Text"=w943, "ActYScl"=0 ("Active Y Scale"), "YScale.NameLbl.Text"=w945, "ActYScl"=1 ("Active Y Scale"), "YScale.Visible"=TRUE ("Y Scale.Visible"), "YScale.NameLbl.Text"=w947) -> ()  [unwired: 2 in, 2 out]
          }
          frame 0 {
            w954 = 0 ("Active X Scale")
            w952 = "" ("X Scale.Name Label.Text")
            n686 = property on="WaveGraph" class="WFGraph (strict)"("ActXScl"=w954, "XScale.NameLbl.Text"=w952, "ActYScl"=w954, "YScale.NameLbl.Text"=w952, "ActYScl"=1 ("Active Y Scale"), "YScale.NameLbl.Text"=w952, "YScale.Visible"=FALSE ("Y Scale.Visible")) -> ()  [unwired: 2 in, 2 out]
          }
          frame 1 {
            n687 = property on="WaveGraph" class="WFGraph (strict)"("ActXScl"=0 ("Active X Scale"), "XScale.NameLbl.Text"=w958, "ActYScl"=0 ("Active Y Scale"), "YScale.NameLbl.Text"=w960, "ActYScl"=1 ("Active Y Scale"), "YScale.Visible"=FALSE ("Y Scale.Visible")) -> ()  [unwired: 2 in, 2 out]
          }
        }
        n688 = property on="Repaint Watermark" class="DigNum (strict)"("Val(Sgnl)"=w893) -> ()  [unwired: 2 in, 2 out]
        n689 = case shown="No Error" w892 {
          frame No Error {
          }
          frame Error {
          }
        }
      }
      event "ColorBox": Value Change {
        # "Graph Color Changing"
        n690 = event-data() -> ("NewVal"=w964:u32)  [unwired: 6 out]
        n691 = local read "OldRow"() -> (w965:i32)
        n692 = local read "Event Name"() -> (w962:string)
        n693 = flat-sequence {
          tunnel: [w975] -> w966
          tunnel: w964 -> [w975]
          tunnel: w965 -> [w974]
          tunnel: w966 -> [w976]
          frame #0 {
            n694 = To Unsigned Long Integer(number=w974) -> (unsigned 32bit integer=w973:u32)
            n695 = property on="Legend" class="MCListbox (strict)"("CellBG"=w975) -> ()  [unwired: 2 in, 2 out]
            n696 = property on="WaveGraph" class="WFGraph (strict)"("Active Plot"=w973) -> (error out=w972:errorcluster)  [unwired: 2 in, 1 out]
            n697 = case shown="No Error" w972 {
              frame No Error {
              }
              frame Error {
              }
            }
          }
          frame #1 {
            n698 = property on="WaveGraph" class="WFGraph (strict)"("Plot.Plot Color"=w976) -> ()  [unwired: 2 in, 2 out]
            n699 = property on="ColorBox" class="ColBox"("Visible"=FALSE) -> ()  [unwired: 2 in, 2 out]
          }
        }
        n700 = call "CRYPreUpdate Sequence.vi"("EventName"="CurLibUpdate") -> ()  [unwired: 15 in]
        n701 = case shown="Default" w962 {
          tunnel: w965 -> [_ w970]
          tunnel: w964 -> [_ w969]
          frame "ViewReport" {
          }
          frame Default {
            n702 = control-ref of="Legend"() -> (w968:refnum<vi>)
            n703 = call "CRYSet Plot Settings.vi"("sAction"="Color", "Color"=w969, "Row"=w970, "Legend Refnum"=w968, "Type"=enum16{"Curves", "Values", "Results", "WFM"}."WFM") -> ()  [unwired: 2 in, 5 out]
          }
        }
      }
      event "ColorBox": Mouse Down {
        n704 = event-data() -> ()  [unwired: 9 out]
        n705 = local read "OldRow"() -> (w981:i32)
        n706 = Bundle By Name(cluster=T5 {"Row"=0, "Column"=0} ("Active Cell:Active Cell"), "Row"=w981, "Column"=1) -> (w978:T5)
        n707 = property on="Legend" class="MCListbox (strict)"("ActiveCell"=w978) -> ()  [unwired: 2 in, 2 out]
      }
      event "WaveGraph": Drag Enter {
        n708 = event-data() -> ("Available Data Names"=w982:string[])  [unwired: 1 out]
        n709 = disable-structure shown="Disabled" {
          disable-tunnel: [w985 TRUE] -> w983
          disable-tunnel: w982 -> [w984 _]
          frame Disabled {
            n710 = Search 1D Array(1D array=w984, element="CRY_GRAPH_DATA") -> (index of element=w987:i32)  [unwired: 1 out]
            n711 = Not Equal?(x=w987, y=-1) -> (x != y?=w985:bool)
          }
          frame Enabled {
          }
        }
        n712 = event-data("Accepted?"=w983) -> ()  [unwired: 1 in, 1 out]
      }
      event "WaveGraph": Drop {
        n713 = event-data() -> ()  [unwired: 2 out]
        n714 = local read "Event Name"() -> (w990:string)
        n715 = local read "TotalPlot"() -> (w995:u32)
        n716 = control-ref of="This VI"() -> (w991:refnum<vi>)
        n717 = call "CRYDrop Data in Same Graph.vi"("pGraph VI"=w991, "Queue"=w992, "Total Plot In"=w995, "sAction"=w990) -> ("Accepted?"=w993:bool, "Total Plot Out"=w994:u32)  [unwired: 3 in, 3 out]
        n718 = local write "TotalPlot"(w994) -> ()
        n719 = event-data("Accepted?"=w993) -> ()  [unwired: 1 in, 1 out]
      }
      event "WaveGraph": Cursor Grab {
        n720 = event-data() -> ("CursIdx"=w996:i32)  [unwired: 1 out]
        n721 = flat-sequence {
          tunnel: w996 -> [w997]
          frame #0 {
            n722 = Equal To 0?(x=w997) -> (x = 0?=w998:bool)
            n723 = local write "NewCursIdx"(w997) -> ()
            n724 = Select(t=u32 1 ("OldCursIdx"), s=w998, f=u32 0 ("OldCursIdx")) -> (s? t:f=w1001:u32)
            n725 = local write "OldCursIdx"(w1001) -> ()
          }
          frame #1 {
            n726 = property on="CursorColor" class="Bool (strict)"("Val(Sgnl)"=TRUE ("Value (Signaling)")) -> ()  [unwired: 2 in, 2 out]
          }
        }
      }
      event "WaveGraph": Cursor Move {
        n727 = event-data() -> ()  [unwired: 10 out]
        n728 = property on="CursorPlot" class="Bool (strict)"("Val(Sgnl)"=TRUE ("Value (Signaling)")) -> ()  [unwired: 2 in, 2 out]
      }
      event "ReportDrop": Value Change {
        n729 = event-data() -> ()  [unwired: 7 out]
        n730 = local read "Event Name"() -> (w1004:string)
        n731 = local read "TotalPlot"() -> (w1008:u32)
        n732 = control-ref of="This VI"() -> (w1006:refnum<vi>)
        n733 = call "CRYDrop Data in Same Graph.vi"("pGraph VI"=w1006, "Queue"=w1005, "Total Plot In"=w1008, "sAction"=w1004) -> ("Total Plot Out"=w1007:u32)  [unwired: 3 in, 4 out]
        n734 = local write "TotalPlot"(w1007) -> ()
      }
      event "WaveGraph": Scale Range Change {
        n735 = event-data() -> ("Kind"=w1010:enum16{"X-Scale", "Y-Scale", "Z-Scale"})  [unwired: 8 out]
        n736 = case shown="\"Y-Scale\"" w1010 {
          frame "X-Scale", Default {
            n737 = property on="WaveGraph" class="WFGraph (strict)"("XScale.ScaleFit"=u8 0 ("X Scale.Scale Fit")) -> ()  [unwired: 2 in, 2 out]
          }
          frame "Y-Scale" {
            n738 = property on="WaveGraph" class="WFGraph (strict)"("YScale.ScaleFit"=u8 0 ("Y Scale.Scale Fit")) -> ()  [unwired: 2 in, 2 out]
            n739 = property on="Repaint Watermark" class="DigNum (strict)"("Val(Sgnl)"=-1 ("y")) -> ()  [unwired: 2 in, 2 out]
          }
        }
        n740 = property on="ScaleRange" class="Bool (strict)"("Val(Sgnl)"=TRUE ("Value (Signaling)")) -> ()  [unwired: 2 in, 2 out]
      }
      event "ScaleRange": Value Change {
        n741 = event-data() -> ()  [unwired: 7 out]
        n742 = local read "PreviewShow"() -> (w1014:bool)
        n743 = case shown="True" w1014 {
          frame False {
          }
          frame True {
            n744 = control-ref of="This VI"() -> (w1015:refnum<vi>)
            n745 = call "CRYScale Change.vi"("Graph VI Ref"=w1015) -> ()  [unwired: 11 in]
          }
        }
      }
      event "Repaint Watermark": Value Change {
        # "Repaint Watermark: 0-none, 1-Unit 1, 2-Unit 1 & 2, -1: surely replot"
        n746 = event-data() -> ("OldVal"=w1021:i32, "NewVal"=w1018:i32)  [unwired: 5 out]
        n747 = Equal?(x=-1 ("y"), y=w1018) -> (x = y?=w1017:bool)
        n748 = case shown="True" w1017 {
          tunnel: w1021 -> [w1024 w1039]
          tunnel: w1018 -> [w1022 _]
          tunnel: [w1023 "Replot" ("PropertyTab")] -> w1020
          tunnel: [w1022 w1039] -> w1016
          frame False {
            n749 = Not Equal?(x=w1024, y=w1022) -> (x != y?=w1025:bool)
            n750 = case shown="True" w1025 {
              tunnel: w1024 -> [_ w1032]
              tunnel: w1022 -> [_ w1031]
              tunnel: [_ w1026] -> w1023
              frame False {
              }
              frame True {
                n751 = Equal To 0?(x=w1032) -> (x = 0?=w1036:bool)
                n752 = Equal?(x=w1031, y=1) -> (x = y?=w1037:bool)
                n753 = Equal?(x=w1032, y=1) -> (x = y?=w1030:bool)
                n754 = Equal To 0?(x=w1031) -> (x = 0?=w1029:bool)
                n755 = And(x=w1030, y=w1029) -> (x .and. y?=w1028:bool)
                n756 = And(x=w1036, y=w1037) -> (x .and. y?=w1034:bool)
                n757 = Or(x=w1034, y=w1028) -> (x .or. y?=w1027:bool)
                n758 = case shown="False" w1027 {
                  tunnel: ["Replot" ("PropertyTab") _] -> w1026
                  frame False {
                  }
                  frame True {
                  }
                }
              }
            }
          }
          frame True {
          }
        }
        n759 = local write "Repaint Watermark"(w1016) -> ()
        n760 = case shown="\"Replot\"" w1020 {
          frame Default {
          }
          frame "Replot" {
            n761 = control-ref of="WaveGraph"() -> (w1042:refnum<vi>)
            n762 = local read "Event Name"() -> (w1041:string)
            n763 = call "CRYPaint WaterMark.vi"("Type"=w1041, "Graph Ref"=w1042) -> ()  [unwired: 10 in]
          }
        }
      }
      event "PreviewGraph": Cursor Move {
        n764 = event-data() -> ("CursIdx"=w1043:i32, "CursLoc"=w1047:cluster{"X":dbl, "Y":dbl})  [unwired: 1 out]
        n765 = property on="PreviewGraph" class="WFGraph (strict)"("ActXScl"=0 ("Active X Scale")) -> ("XScale.Maximum"=w1044:dbl, "XScale.Minimum"=w1045:dbl)  [unwired: 2 in, 2 out]
        n766 = property on="WaveGraph" class="WFGraph (strict)"("ActXScl"=0 ("Active X Scale"), "XScale.ScaleFit"=u8 0 ("X Scale.Scale Fit")) -> ()  [unwired: 2 in, 2 out]
        n767 = Unbundle By Name(w1047) -> ("X"=w1053:dbl)
        n768 = Less Or Equal?(x=w1053, y=w1045) -> (x <= y?=w1049:bool)
        n769 = Greater Or Equal?(x=w1053, y=w1044) -> (x >= y?=w1050:bool)
        n770 = Or(x=w1049, y=w1050) -> (x .or. y?=w1048:bool)
        n771 = case shown="True" w1048 {
          tunnel: w1049 -> [_ w1101]
          tunnel: w1043 -> [_ w1096]
          frame False {
            n772 = property on="PreviewGraph" class="WFGraph (strict)"("Active Cursor"=u32 0, "Active Cursor"=u32 1) -> ("Cursor.Cursor X"=w1074:dbl, "Cursor.Cursor X"=w1075:dbl)  [unwired: 2 in, 2 out]
            n773 = property on="PreviewGraph" class="WFGraph (strict)"("ActXScl"=0 ("Active X Scale")) -> ("XScale.Maximum"=w1068:dbl, "XScale.Minimum"=w1067:dbl)  [unwired: 2 in, 2 out]
            n774 = control-ref of="This VI"() -> (w1057:refnum<vi>)
            n775 = property on="WaveGraph" class="WFGraph (strict)"("ActXScl"=0 ("Active X Scale"), "XScale.ScaleFit"=u8 0 ("X Scale.Scale Fit")) -> (error out=w1058:errorcluster)  [unwired: 2 in, 1 out]
            n776 = Greater?(x=w1074, y=w1075) -> (0:w1073:bool)
            n777 = case shown="True" w1073 {
              tunnel: w1074 -> [w1093 w1095]
              tunnel: w1075 -> [w1092 w1094]
              tunnel: [w1093 w1094] -> w1061
              tunnel: [w1092 w1095] -> w1069
              frame False {
              }
              frame True {
              }
            }
            n778 = call "CRYPlot Wave Graph Preview.vi"("sOption"="Move", "Graph VI Ref"=w1057) -> ()  [unwired: 10 in]
            n779 = Subtract(x=w1068, y=w1067) -> (x-y=w1063:dbl)
            n780 = property on="WaveGraph" class="WFGraph (strict)"(error in=w1058, "XScale.Minimum"=w1061, "XScale.Maximum"=w1069) -> ()  [unwired: 1 in, 2 out]
            n781 = Subtract(x=w1061, y=w1067) -> (x-y=w1066:dbl)
            n782 = Subtract(x=w1069, y=w1067) -> (x-y=w1064:dbl)
            n783 = Divide(x=w1066, y=w1063) -> (x/y=w1065:dbl)
            n784 = Divide(x=w1064, y=w1063) -> (x/y=w1062:dbl)
            n785 = Subtract(x=w1065, y=w1062) -> (x-y=w1054:dbl)
            n786 = Equal To 0?(x=w1054) -> (x = 0?=w1055:bool)
            n787 = case shown="False" w1055 {
              tunnel: w1054 -> [w1080 _]
              tunnel: w1065 -> [w1076 _]
              frame False {
                n788 = property on="Scrollbar" class="Scroll (strict)"() -> ("DocMax"=w1082:dbl, "PageSize"=w1089:dbl)  [unwired: 2 in, 2 out]
                n789 = Divide(x=w1089, y=w1080) -> (x/y=w1079:dbl)
                n790 = local read "ScaleMax"() -> (w1078:dbl)
                n791 = local read "ScaleMin"() -> (w1077:dbl)
                n792 = Add(x=w1082, y=w1079) -> (x+y=w1081:dbl)
                n793 = property on="Scrollbar" class="Scroll (strict)"("DocMin"=w1081) -> ("DocMax"=w1091:dbl, "DocMin"=w1090:dbl)  [unwired: 2 in, 2 out]
                n794 = Subtract(x=w1078, y=w1077) -> (x-y=w1086:dbl)
                n795 = Subtract(x=w1076, y=w1077) -> (x-y=w1083:dbl)
                n796 = Subtract(x=w1091, y=w1090) -> (x-y=w1084:dbl)
                n797 = Multiply(x=w1083, y=w1084) -> (x*y=w1085:dbl)
                n798 = Divide(x=w1085, y=w1086) -> (x/y=w1087:dbl)
                n799 = Add(x=w1087, y=w1090) -> (x+y=w1088:dbl)
                n800 = property on="Scrollbar" class="Scroll (strict)"("Value"=w1088) -> ()  [unwired: 2 in, 2 out]
              }
              frame True {
              }
            }
          }
          frame True {
            n801 = property on="PreviewGraph" class="WFGraph (strict)"("ActXScl"=0 ("Active X Scale")) -> ("XScale.Maximum"=w1099:dbl, "XScale.Minimum"=w1100:dbl)  [unwired: 2 in, 2 out]
            n802 = Subtract(x=w1099, y=w1100) -> (x-y=w1102:dbl)
            n803 = case shown="True" w1101 {
              tunnel: w1100 -> [w1109 _]
              tunnel: w1099 -> [_ w1112]
              tunnel: [w1108 w1111] -> w1098
              tunnel: w1096 -> [w1107 w1110]
              frame True {
                n804 = property on="PreviewGraph" class="WFGraph (strict)"("Active Cursor"=w1107, "Cursor.Cursor X"=w1109) -> (error out=w1108:errorcluster)  [unwired: 2 in, 1 out]
              }
              frame False {
                n805 = property on="PreviewGraph" class="WFGraph (strict)"("Active Cursor"=w1110, "Cursor.Cursor X"=w1112) -> (error out=w1111:errorcluster)  [unwired: 2 in, 1 out]
              }
            }
            n806 = flat-sequence {
              tunnel: w1100 -> [w1119]
              tunnel: w1102 -> [w1116]
              tunnel: w1097 -> [w1113]
              frame #0 {
                n807 = property on="PreviewGraph" class="WFGraph (strict)"(error in=w1113, "Active Cursor"=u32 0, "Active Cursor"=u32 1) -> ("Cursor.Cursor X"=w1123:dbl, "Cursor.Cursor X"=w1122:dbl)  [unwired: 1 in, 2 out]
                n808 = Greater?(x=w1123, y=w1122) -> (0:w1139:bool)
                n809 = case shown="True" w1139 {
                  tunnel: w1123 -> [w1143 w1145]
                  tunnel: w1122 -> [w1142 w1144]
                  tunnel: [w1143 w1144] -> w1121
                  tunnel: [w1142 w1145] -> w1120
                  frame False {
                  }
                  frame True {
                  }
                }
                n810 = Subtract(x=w1121, y=w1119) -> (x-y=w1118:dbl)
                n811 = Subtract(x=w1120, y=w1119) -> (x-y=w1115:dbl)
                n812 = Divide(x=w1118, y=w1116) -> (x/y=w1117:dbl)
                n813 = Divide(x=w1115, y=w1116) -> (x/y=w1114:dbl)
                n814 = property on="WaveGraph" class="WFGraph (strict)"("XScale.Minimum"=w1121, "XScale.Maximum"=w1120) -> ()  [unwired: 2 in, 2 out]
                n815 = property on="Scrollbar" class="Scroll (strict)"() -> ("DocMax"=w1133:dbl, "PageSize"=w1126:dbl)  [unwired: 2 in, 2 out]
                n816 = Subtract(x=w1117, y=w1114) -> (x-y=w1135:dbl)
                n817 = local read "ScaleMax"() -> (w1137:dbl)
                n818 = local read "ScaleMin"() -> (w1138:dbl)
                n819 = Divide(x=w1126, y=w1135) -> (x/y=w1136:dbl)
                n820 = Add(x=w1133, y=w1136) -> (x+y=w1134:dbl)
                n821 = property on="Scrollbar" class="Scroll (strict)"("DocMin"=w1134) -> ("DocMax"=w1124:dbl, "DocMin"=w1125:dbl)  [unwired: 2 in, 2 out]
                n822 = Subtract(x=w1137, y=w1138) -> (x-y=w1129:dbl)
                n823 = Subtract(x=w1117, y=w1138) -> (x-y=w1132:dbl)
                n824 = Subtract(x=w1124, y=w1125) -> (x-y=w1131:dbl)
                n825 = Multiply(x=w1132, y=w1131) -> (x*y=w1130:dbl)
                n826 = Divide(x=w1130, y=w1129) -> (x/y=w1128:dbl)
                n827 = Add(x=w1128, y=w1125) -> (x+y=w1127:dbl)
                n828 = property on="Scrollbar" class="Scroll (strict)"("Value"=w1127) -> ()  [unwired: 2 in, 2 out]
              }
            }
            n829 = flat-sequence {
              tunnel: w1098 -> [w1104]
              tunnel: [w1104] -> w1097
              frame #0 {
                n830 = control-ref of="This VI"() -> (w1106:refnum<vi>)
                n831 = call "CRYPlot Wave Graph Preview.vi"("sOption"="Move", "Graph VI Ref"=w1106) -> ()  [unwired: 10 in]
              }
            }
          }
        }
      }
      event "PreviewGraph": Mouse Down {
        n832 = event-data() -> ("Button"=w1146:u16, "Coords"=w1147:T1)  [unwired: 1 out]
        n833 = case shown="2" w1146 {
          tunnel: w1147 -> [w1159 w1286]
          frame Default {
            n834 = property on="PreviewGraph" class="WFGraph (strict)"() -> ("Plot Bounds"=w1160:T6, "Width"=w1158:u32)  [unwired: 2 in, 2 out]
            n835 = property on="WaveGraph" class="WFGraph (strict)"("ActXScl"=0 ("Active X Scale"), "XScale.ScaleFit"=u8 0 ("X Scale.Scale Fit")) -> ()  [unwired: 2 in, 2 out]
            n836 = Unbundle By Name(w1159) -> ("Horizontal"=w1156:i32)
            n837 = To Long Integer(number=w1158) -> (32bit integer=w1153:i32)
            n838 = Unbundle By Name(w1160) -> ("Left"=w1157:i16)
            n839 = To Long Integer(number=w1157) -> (32bit integer=w1154:i32)
            n840 = Add(x=w1154, y=w1153) -> (x+y=w1155:i32)
            n841 = Less?(x=w1156, y=w1154) -> (x < y?=w1149:bool)
            n842 = Greater?(x=w1156, y=w1155) -> (0:w1150:bool)
            n843 = Or(x=w1149, y=w1150) -> (x .or. y?=w1148:bool)
            n844 = case shown="False" w1148 {
              tunnel: w1154 -> [w1165 _]
              tunnel: w1153 -> [w1164 _]
              tunnel: w1156 -> [w1163 _]
              tunnel: w1149 -> [_ w1239]
              frame False {
                n845 = property on="PreviewGraph" class="WFGraph (strict)"("ActXScl"=0 ("Active X Scale")) -> ("XScale.Maximum"=w1175:dbl, "XScale.Minimum"=w1171:dbl)  [unwired: 2 in, 2 out]
                n846 = property on="PreviewGraph" class="WFGraph (strict)"("Active Cursor"=u32 0, "Active Cursor"=u32 1) -> ("Cursor.Cursor X"=w1162:dbl, "Cursor.Cursor X"=w1161:dbl)  [unwired: 2 in, 2 out]
                n847 = Subtract(x=w1163, y=w1165) -> (x-y=w1178:i32)
                n848 = Divide(x=w1178, y=w1164) -> (x/y=w1174:dbl)
                n849 = Subtract(x=w1175, y=w1171) -> (x-y=w1170:dbl)
                n850 = Less Or Equal?(x=w1162, y=w1161) -> (x <= y?=w1182:bool)
                n851 = Multiply(x=w1174, y=w1170) -> (x*y=w1173:dbl)
                n852 = Subtract(x=w1162, y=w1161) -> (x-y=w1169:dbl)
                n853 = flat-sequence {
                  tunnel: w1183 -> [_]
                  tunnel: w1171 -> [w1189]
                  tunnel: w1170 -> [w1186]
                  frame #0 {
                    n854 = property on="PreviewGraph" class="WFGraph (strict)"("Active Cursor"=u32 0, "Active Cursor"=u32 1) -> ("Cursor.Cursor X"=w1193:dbl, "Cursor.Cursor X"=w1192:dbl)  [unwired: 2 in, 2 out]
                    n855 = Greater?(x=w1193, y=w1192) -> (0:w1209:bool)
                    n856 = case shown="True" w1209 {
                      tunnel: w1193 -> [w1213 w1215]
                      tunnel: w1192 -> [w1212 w1214]
                      tunnel: [w1213 w1214] -> w1191
                      tunnel: [w1212 w1215] -> w1190
                      frame False {
                      }
                      frame True {
                      }
                    }
                    n857 = Subtract(x=w1191, y=w1189) -> (x-y=w1188:dbl)
                    n858 = Subtract(x=w1190, y=w1189) -> (x-y=w1185:dbl)
                    n859 = Divide(x=w1188, y=w1186) -> (x/y=w1187:dbl)
                    n860 = Divide(x=w1185, y=w1186) -> (x/y=w1184:dbl)
                    n861 = property on="WaveGraph" class="WFGraph (strict)"("XScale.Minimum"=w1191, "XScale.Maximum"=w1190) -> ()  [unwired: 2 in, 2 out]
                    n862 = property on="Scrollbar" class="Scroll (strict)"() -> ("DocMax"=w1203:dbl, "PageSize"=w1196:dbl)  [unwired: 2 in, 2 out]
                    n863 = Subtract(x=w1187, y=w1184) -> (x-y=w1205:dbl)
                    n864 = local read "ScaleMax"() -> (w1207:dbl)
                    n865 = local read "ScaleMin"() -> (w1208:dbl)
                    n866 = Divide(x=w1196, y=w1205) -> (x/y=w1206:dbl)
                    n867 = Add(x=w1203, y=w1206) -> (x+y=w1204:dbl)
                    n868 = property on="Scrollbar" class="Scroll (strict)"("DocMin"=w1204) -> ("DocMax"=w1194:dbl, "DocMin"=w1195:dbl)  [unwired: 2 in, 2 out]
                    n869 = Subtract(x=w1207, y=w1208) -> (x-y=w1199:dbl)
                    n870 = Subtract(x=w1187, y=w1208) -> (x-y=w1202:dbl)
                    n871 = Subtract(x=w1194, y=w1195) -> (x-y=w1201:dbl)
                    n872 = Multiply(x=w1202, y=w1201) -> (x*y=w1200:dbl)
                    n873 = Divide(x=w1200, y=w1199) -> (x/y=w1198:dbl)
                    n874 = Add(x=w1198, y=w1195) -> (x+y=w1197:dbl)
                    n875 = property on="Scrollbar" class="Scroll (strict)"("Value"=w1197) -> ()  [unwired: 2 in, 2 out]
                  }
                }
                n876 = Absolute Value(x=w1169) -> (abs(x)=w1168:dbl)
                n877 = Add(x=w1173, y=w1171) -> (x+y=w1172:dbl)
                n878 = Divide(x=w1168, y=2.0) -> (x/y=w1166:dbl)
                n879 = case shown="True" w1182 {
                  tunnel: [w1220 w1228] -> w1180
                  tunnel: w1172 -> [w1216 w1225]
                  tunnel: w1162 -> [w1219 _]
                  tunnel: w1161 -> [_ w1224]
                  tunnel: w1166 -> [w1218 w1227]
                  frame True {
                    n880 = Add(x=w1219, y=w1218) -> (x+y=w1217:dbl)
                    n881 = Greater?(x=w1217, y=w1216) -> (0:w1223:bool)
                    n882 = Select(t=u32 0 ("Active Cursor"), s=w1223, f=u32 1) -> (s? t:f=w1220:u32)
                  }
                  frame False {
                    n883 = Add(x=w1224, y=w1227) -> (x+y=w1226:dbl)
                    n884 = Greater?(x=w1226, y=w1225) -> (0:w1231:bool)
                    n885 = Select(t=u32 1 ("Active Cursor"), s=w1231, f=u32 0) -> (s? t:f=w1228:u32)
                  }
                }
                n886 = property on="PreviewGraph" class="WFGraph (strict)"("Active Cursor"=w1180, "Cursor.Cursor X"=w1172) -> (error out=w1179:errorcluster)  [unwired: 2 in, 1 out]
                n887 = flat-sequence {
                  tunnel: w1179 -> [w1234]
                  tunnel: [w1234] -> w1183
                  frame #0 {
                    n888 = control-ref of="This VI"() -> (w1233:refnum<vi>)
                    n889 = call "CRYPlot Wave Graph Preview.vi"("sOption"="Move", "Graph VI Ref"=w1233) -> ()  [unwired: 10 in]
                  }
                }
              }
              frame True {
                n890 = property on="PreviewGraph" class="WFGraph (strict)"("ActXScl"=0 ("Active X Scale")) -> ("XScale.Maximum"=w1237:dbl, "XScale.Minimum"=w1238:dbl)  [unwired: 2 in, 2 out]
                n891 = Subtract(x=w1237, y=w1238) -> (x-y=w1240:dbl)
                n892 = case shown="True" w1239 {
                  tunnel: w1238 -> [w1246 _]
                  tunnel: w1237 -> [_ w1250]
                  tunnel: [w1245 w1249] -> w1236
                  frame True {
                    n893 = property on="PreviewGraph" class="WFGraph (strict)"("Active Cursor"=u32 0, "Cursor.Cursor X"=w1246, "Active Cursor"=u32 1, "Cursor.Cursor X"=w1246) -> (error out=w1245:errorcluster)  [unwired: 2 in, 1 out]
                  }
                  frame False {
                    n894 = property on="PreviewGraph" class="WFGraph (strict)"("Active Cursor"=u32 0, "Cursor.Cursor X"=w1250, "Active Cursor"=u32 1, "Cursor.Cursor X"=w1250) -> (error out=w1249:errorcluster)  [unwired: 2 in, 1 out]
                  }
                }
                n895 = flat-sequence {
                  tunnel: w1238 -> [w1259]
                  tunnel: w1240 -> [w1256]
                  tunnel: w1235 -> [w1253]
                  frame #0 {
                    n896 = property on="PreviewGraph" class="WFGraph (strict)"(error in=w1253, "Active Cursor"=u32 0, "Active Cursor"=u32 1) -> ("Cursor.Cursor X"=w1263:dbl, "Cursor.Cursor X"=w1262:dbl)  [unwired: 1 in, 2 out]
                    n897 = Greater?(x=w1263, y=w1262) -> (0:w1279:bool)
                    n898 = case shown="True" w1279 {
                      tunnel: w1263 -> [w1283 w1285]
                      tunnel: w1262 -> [w1282 w1284]
                      tunnel: [w1283 w1284] -> w1261
                      tunnel: [w1282 w1285] -> w1260
                      frame False {
                      }
                      frame True {
                      }
                    }
                    n899 = Subtract(x=w1261, y=w1259) -> (x-y=w1258:dbl)
                    n900 = Subtract(x=w1260, y=w1259) -> (x-y=w1255:dbl)
                    n901 = Divide(x=w1258, y=w1256) -> (x/y=w1257:dbl)
                    n902 = Divide(x=w1255, y=w1256) -> (x/y=w1254:dbl)
                    n903 = property on="WaveGraph" class="WFGraph (strict)"("XScale.Minimum"=w1261, "XScale.Maximum"=w1260) -> ()  [unwired: 2 in, 2 out]
                    n904 = property on="Scrollbar" class="Scroll (strict)"() -> ("DocMax"=w1273:dbl, "PageSize"=w1266:dbl)  [unwired: 2 in, 2 out]
                    n905 = Subtract(x=w1257, y=w1254) -> (x-y=w1275:dbl)
                    n906 = local read "ScaleMax"() -> (w1277:dbl)
                    n907 = local read "ScaleMin"() -> (w1278:dbl)
                    n908 = Divide(x=w1266, y=w1275) -> (x/y=w1276:dbl)
                    n909 = Add(x=w1273, y=w1276) -> (x+y=w1274:dbl)
                    n910 = property on="Scrollbar" class="Scroll (strict)"("DocMin"=w1274) -> ("DocMax"=w1264:dbl, "DocMin"=w1265:dbl)  [unwired: 2 in, 2 out]
                    n911 = Subtract(x=w1277, y=w1278) -> (x-y=w1269:dbl)
                    n912 = Subtract(x=w1257, y=w1278) -> (x-y=w1272:dbl)
                    n913 = Subtract(x=w1264, y=w1265) -> (x-y=w1271:dbl)
                    n914 = Multiply(x=w1272, y=w1271) -> (x*y=w1270:dbl)
                    n915 = Divide(x=w1270, y=w1269) -> (x/y=w1268:dbl)
                    n916 = Add(x=w1268, y=w1265) -> (x+y=w1267:dbl)
                    n917 = property on="Scrollbar" class="Scroll (strict)"("Value"=w1267) -> ()  [unwired: 2 in, 2 out]
                  }
                }
                n918 = flat-sequence {
                  tunnel: w1236 -> [w1242]
                  tunnel: [w1242] -> w1235
                  frame #0 {
                    n919 = control-ref of="This VI"() -> (w1244:refnum<vi>)
                    n920 = call "CRYPlot Wave Graph Preview.vi"("sOption"="Move", "Graph VI Ref"=w1244) -> ()  [unwired: 10 in]
                  }
                }
              }
            }
          }
          frame 2 {
            n921 = local write "PreviewCoords"(w1286) -> ()
          }
        }
      }
      event "PreviewShow": Value Change {
        n922 = event-data() -> ("NewVal"=w1287:bool)  [unwired: 6 out]
        n923 = flat-sequence {
          tunnel: w1287 -> [w1292]
          frame #0 {
            n924 = Select(t="DA_PRE_VIEW", s=w1292, f="DA_PRE_HIDE") -> (s? t:f=w1291:string)
            n925 = control-ref of="This VI"() -> (w1288:refnum<vi>)
            n926 = call "CRYPreview InsDel.vi"("Graph VI Ref"=w1288, "sAction"=w1291) -> ()  [unwired: 10 in]
          }
          frame #1 {
            n927 = property on="ToolbarUpdate" class="Bool (strict)"("Val(Sgnl)"=TRUE ("Value (Signaling)")) -> ()  [unwired: 2 in, 2 out]
          }
        }
      }
      event "PreviewGraph": Scale Range Change {
        n928 = event-data() -> ("NewRange"=w1301:T10)  [unwired: 8 out]
        n929 = disable-structure shown="Disabled" {
          frame Disabled {
            n930 = property on="WaveGraph" class="WFGraph (strict)"("ActXScl"=0 ("Active X Scale"), "XScale.ScaleFit"=u8 0 ("X Scale.Scale Fit")) -> ()  [unwired: 2 in, 2 out]
          }
          frame Enabled {
          }
        }
        n931 = local read "PreviewScaleMax"() -> (w1294:dbl)
        n932 = local read "PreviewScaleMin"() -> (w1295:dbl)
        n933 = Unbundle By Name(w1301) -> ("Minimum"=w1300:dbl, "Maximum"=w1299:dbl)
        n934 = Less?(x=w1300, y=w1295) -> (x < y?=w1298:bool)
        n935 = Greater?(x=w1299, y=w1294) -> (0:w1297:bool)
        n936 = Or(x=w1298, y=w1297) -> (x .or. y?=w1296:bool)
        n937 = case shown="True" w1296 {
          tunnel: w1295 -> [_ w1306]
          tunnel: w1294 -> [_ w1305]
          frame False {
          }
          frame True {
            n938 = property on="PreviewGraph" class="WFGraph (strict)"("ActXScl"=0 ("Active X Scale"), "XScale.Maximum"=w1305, "XScale.Minimum"=w1306) -> (error out=w1304:errorcluster)  [unwired: 2 in, 1 out]
            n939 = property on="ScaleRange" class="Bool (strict)"(error in=w1304, "Val(Sgnl)"=TRUE ("Value (Signaling)")) -> ()  [unwired: 1 in, 2 out]
          }
        }
      }
      event "Scrollbar": Value Change {
        n940 = event-data() -> ("NewVal"=w1324:dbl)  [unwired: 6 out]
        n941 = local read "ScaleMax"() -> (w1334:dbl)
        n942 = local read "ScaleMin"() -> (w1335:dbl)
        n943 = property on="Scrollbar" class="Scroll (strict)"() -> ("DocMin"=w1333:dbl, "DocMax"=w1332:dbl)  [unwired: 2 in, 2 out]
        n944 = property on="PreviewGraph" class="WFGraph (strict)"("Active Cursor"=u32 0, "Active Cursor"=u32 1) -> ("Cursor.Cursor X"=w1327:dbl, "Cursor.Cursor X"=w1328:dbl)  [unwired: 2 in, 2 out]
        n945 = property on="WaveGraph" class="WFGraph (strict)"("ActXScl"=0 ("Active X Scale"), "XScale.ScaleFit"=u8 0 ("X Scale.Scale Fit")) -> (error out=w1309:errorcluster)  [unwired: 2 in, 1 out]
        n946 = property on="PreviewGraph" class="WFGraph (strict)"(error in=w1309, "ActXScl"=0 ("Active X Scale")) -> ("XScale.Maximum"=w1320:dbl, "XScale.Minimum"=w1315:dbl)  [unwired: 1 in, 2 out]
        n947 = Subtract(x=w1332, y=w1333) -> (x-y=w1339:dbl)
        n948 = Subtract(x=w1334, y=w1335) -> (x-y=w1337:dbl)
        n949 = Subtract(x=w1324, y=w1333) -> (x-y=w1336:dbl)
        n950 = Subtract(x=w1327, y=w1328) -> (x-y=w1329:dbl)
        n951 = Multiply(x=w1336, y=w1337) -> (x*y=w1338:dbl)
        n952 = Subtract(x=w1320, y=w1315) -> (x-y=w1313:dbl)
        n953 = Absolute Value(x=w1329) -> (abs(x)=w1314:dbl)
        n954 = Divide(x=w1338, y=w1339) -> (x/y=w1319:dbl)
        n955 = Divide(x=w1314, y=w1313) -> (x/y=w1312:dbl)
        n956 = Less Or Equal To 0?(x=w1329) -> (x <= 0?=w1330:bool)
        n957 = Add(x=w1312, y=w1319) -> (x+y=w1318:dbl)
        n958 = Multiply(x=w1313, y=w1319) -> (x*y=w1316:dbl)
        n959 = Multiply(x=w1313, y=w1318) -> (x*y=w1317:dbl)
        n960 = Add(x=w1315, y=w1317) -> (x+y=w1322:dbl)
        n961 = Add(x=w1315, y=w1316) -> (x+y=w1321:dbl)
        n962 = case shown="False" w1330 {
          tunnel: w1321 -> [w1343 w1348]
          tunnel: w1322 -> [w1342 w1347]
          tunnel: [w1344 w1349] -> w1331
          tunnel: [w1343 w1348] -> w1340
          tunnel: [w1342 w1347] -> w1341
          frame True {
            n963 = property on="PreviewGraph" class="WFGraph (strict)"("Active Cursor"=u32 0, "Cursor.Cursor X"=w1343, "Active Cursor"=u32 1, "Cursor.Cursor X"=w1342) -> (error out=w1344:errorcluster)  [unwired: 2 in, 1 out]
          }
          frame False {
            n964 = property on="PreviewGraph" class="WFGraph (strict)"("Active Cursor"=u32 1, "Cursor.Cursor X"=w1348, "Active Cursor"=u32 0, "Cursor.Cursor X"=w1347) -> (error out=w1349:errorcluster)  [unwired: 2 in, 1 out]
          }
        }
        n965 = property on="WaveGraph" class="WFGraph (strict)"("XScale.Minimum"=w1340, "XScale.Maximum"=w1341) -> ()  [unwired: 2 in, 2 out]
        n966 = flat-sequence {
          tunnel: w1331 -> [_]
          frame #0 {
            n967 = control-ref of="This VI"() -> (w1353:refnum<vi>)
            n968 = call "CRYPlot Wave Graph Preview.vi"("sOption"="Move", "Graph VI Ref"=w1353) -> ()  [unwired: 10 in]
          }
        }
      }
      event "OpenProperty": Value Change {
        n969 = event-data() -> ()  [unwired: 7 out]
        n970 = flat-sequence {
          frame #0 {
            n971 = local read "PropertyTab"() -> (w1354:string)
            n972 = control-ref of="This VI"() -> (w1355:refnum<vi>)
            n973 = call "CRYGraph Property Window Main.vi"("TabName"=w1354, "pGraph VI In"=w1355) -> ()  [unwired: 1 in, 9 out]
          }
          frame #1 {
            n974 = local write "PropertyTab"("" ("PropertyTab")) -> ()
          }
        }
      }
      event "ToolbarUpdate": Value Change {
        n975 = event-data() -> ()  [unwired: 7 out]
        n976 = local read "Test"() -> (w1357:string)
        n977 = case shown="Default" w1357 {
          frame "Test" {
          }
          frame Default {
            n978 = local read "Event Name"() -> (w1358:string)
            n979 = case shown="Default" w1358 {
              frame "ViewReport" {
              }
              frame Default {
                n980 = control-ref of="This VI"() -> (w1360:refnum<vi>)
                n981 = call "CRYPreUpdate Sequence.vi"("EventName"="CurLibUpdate") -> ()  [unwired: 15 in]
                n982 = call "CRYUpdate DataView Toolbar.vi"("pVI"=w1360) -> ()  [unwired: 11 in]
              }
            }
          }
        }
      }
    }
    n983 = global read "CRYMain Sub Window Global.vi" "gStop"() -> (w207:bool)
    n984 = Or(x=w207, y="stop") -> (x .or. y?=w203:bool)
  }
  n985 = Release Queue(queue=w7, error in (no error)=w10) -> (error out=w8:errorcluster)  [unwired: 3 out]
  n986 = flat-sequence {
    tunnel: w12 -> [_]
    tunnel: w8 -> [_]
    frame #0 {
      n987 = local write "StateOut"(TRUE ("StateOut")) -> ()
    }
  }
